vi "TI sbRIO Main (FPGA) old.vi"() -> ()   [LabVIEW 2019]
uses:
  <userlib>/_NI SPI IP/FPGA/Controllers/Public/Transfer Settings.ctl
  Type Defs/Diagnostic Mode.ctl
  Controls/SPI Channels.ctl
  <vilib>/Platform/TimedLoop/XDataNode/timing_clust.ctl
  <vilib>/Platform/TimedLoop/XDataNode/nitl_modes.ctl
  <vilib>/Platform/TimedLoop/XDataNode/wakeup.ctl
  <vilib>/rvi/FXPMathLib/FxpDiv/subVIs/nifxpmath_Div_SimConfig.ctl
  <vilib>/rvi/FXPMathLib/basic elements/FxpIntAccumulator/subVIs/nifxpmath_IntAccumulator_SimConfig.ctl
  <vilib>/rvi/FXPMathLib/FxpSqrt/subVIs/nifxpmath_Sqrt_SimConfig.ctl
  <vilib>/fxp/LVFixedPointOverflowPolicyTypeDef.ctl
  <userlib>/_NI SPI IP/FPGA/Controllers/Public/Spi Master Inputs.ctl
  <vilib>/rvi/Emulation/niFpgaGetClockAttributes.vi
  <vilib>/rvi/Emulation/niFpgaSctlEmulationGetInTimedLoop.vi
  <vilib>/rvi/Emulation/niFpgaEmulationReportErrorSimple.vi
  <vilib>/rvi/eio/common/nirviEmuTemplateMethod_errors.vi
  Onboard AIs Global.vi
  <vilib>/rvi/Emulation/niFpgaProcessEmulError.vi
  <vilib>/rvi/Emulation/niFpgaCriticalErrorInLSC.vi
  ADC AI Global.vi
  <vilib>/rvi/FXPMathLib/FxpDiv/simVIs/DllFxpDivTemp_sub.vi
  <vilib>/rvi/DataTransferAndStorage/Container/Common/niFpgaContainerExecOnDevCompGetState.vi
  <vilib>/rvi/Emulation/niFpgaEmulationIsFPGAContextNoSignature.vi
  <vilib>/rvi/errors/niFpgaSetErrorForExecOnDevCompSimple.vi
  <vilib>/rvi/eio/common/nirviEmuReportErrorAndStop.vi
  <vilib>/rvi/DataTransferAndStorage/Container/Common/niFpgaContainerGetUniqueNameForEmu.vi
  <vilib>/rvi/FIFO/Fifo_Resource/nirvififoEmulationSetSize.vi
  <vilib>/rvi/FIFO/Fifo_Resource/nirviFifoEmulationQueueMgr.vi
  <instcachedir>/0/nirviFifoEmulationQueueMgr_E5CAEC123FF24DC58D834DCA3CDAA9B5.lvgen/nirviFifoEmulationQueueMgr_E5CAEC123FF24DC58D834DCA3CDAA9B5_000.vi
  <vilib>/rvi/FIFO/Fifo_Resource/nirvififoEmulationDetermineInputValidOut.vi
  <vilib>/rvi/FIFO/Fifo_Resource/nirvififoEmulationCreateLock.vi
  <vilib>/rvi/FIFO/Fifo_Resource/nirvififoEmulationObtainLock.vi
  <vilib>/rvi/FIFO/Fifo_Resource/nirvififoEmulationReleaseLock.vi
  <vilib>/rvi/occurrence/nirviWaitOnOccurrenceBase.vi
  <vilib>/rvi/errors/nirviReportUnexpectedCaseInternalError.vi
  <vilib>/rvi/errors/nirviReportUnexpectedCaseInternalError (U32).vi
  <vilib>/Utility/error.llb/Clear Errors.vi
  <vilib>/rvi/interface/RandomDataEmulation/niFpgaRandomDataHandleErrors.vi
  Diagnostic Global.vi
  Diagnostic Global (U32).vi
  Flow Frequencies Global.vi
  ADC AI Global (Avg).vi
  <vilib>/rvi/Analysis/common/codeGenErrors/XNode/niFpgaXNodeCodeGenErrorHandle.vi
  <vilib>/rvi/FXPMathLib/basic elements/FxpIntAccumulator/simVIs/DllFxpIntAccumulator_sub.vi
  <vilib>/rvi/FXPMathLib/FxpSqrt/simVIs/DllSqrtTemp_sub.vi
  Pump Currents Global.vi
  ADC AI Global (U32).vi
  <vilib>/eio/EIONode/EIONode.xnode
  <vilib>/rvi/FXPMathLib/FxpDiv/XNode/nifxpmath_Div.xnode
  <vilib>/rvi/DataTransferAndStorage/Container/XNode/niFpgaContainer.xnode
  <vilib>/rvi/FIFO/Fifo_Resource/niFpgaFifoEmulationRefIn.vi
  <vilib>/rvi/FXPMathLib/FxpMul/XNode/nifxpmath_Multiplier.xnode
  <vilib>/rvi/FXPMathLib/FxpAdd/XNode/nifxpmath_Add.xnode
  <vilib>/rvi/Analysis/measure/butterworth/XNode/niFpgaButterworthFilter.xnode
  <vilib>/rvi/Analysis/measure/dc-rms/XNode/niFpgaDC-RMS.xnode
  <vilib>/Platform/TimedLoop/XDataNode/XDataNode.xnode
  <vilib>/rvi/FXPMathLib/basic elements/FxpIntAccumulator/XNode/nifxpmath_IntAccumulator.xnode
  <vilib>/rvi/FXPMathLib/FxpSqrt/XNode/nifxpmath_Sqrt.xnode
  <vilib>/eio/EIOMethodNode/EIOMethodNode.xnode
  <vilib>/rvi/interface/RandomDataEmulation/nirviRandomDataFpgaReadWriteTemplate.vi
  <vilib>/rvi/FXPMathLib/sim/FxpSim.dll
  <vilib>/Platform/TimedLoop/XDataNode/XDNodeRunTimeDep.lvlib
  <userlib>/_NI SPI IP/FPGA/Controllers/NI SPI IP FPGA.lvlib
panel:
  in  "PWM Freq":fxp<+,32,0>=2.499902620911598e-06 caption="frequency (periods/tick)"
  in  "PWM Duty":fxp<+,32,0>[](array[numeric])=[0.0, 0.0, 0.0, 0.0, 0.0, 0.0]
  out "Pump Cmds":fxp<+/-,28,17>[](array[numeric])
  in  "Pumps Present":bool[](array[boolean])=[FALSE, FALSE, FALSE, FALSE, FALSE, FALSE]
  in  "Pump Cmds (Duty)":u32[](array[numeric])=[0, 0, 0, 0, 0, 0]
  in  "Debug Restarts":bool
  out "Pump No Starts":u32[](array[numeric])
  in  "Initial No Starts":u32[](array[numeric])=[0, 0, 0, 0, 0, 0]
  in  "Pump Start Time":u32
  out "Restarts":i32[](array[numeric])
  out "Cmd Pump Starts":u32[](array[numeric])
  in  "Stop Command":fxp<+,32,0>
  in  "Initial Cmd Starts":u32[](array[numeric])=[0, 0, 0, 0, 0, 0]
  in  "Ctrl Currents":fxp<+/-,28,17>[](array[numeric])=[0.0, 0.0, 0.0, 0.0, 0.0, 0.0]
  in  "Initial Acutal Starts":u32[](array[numeric])=[0, 0, 0, 0, 0, 0]
  in  "Power Relays":bool[](array[boolean])=[FALSE, FALSE, FALSE, FALSE, FALSE, FALSE]
  out "Actual Pump Starts":u32[](array[numeric])
  out "Timers (ms)":u32[](array[numeric])
  out "Pump On States":bool[](array[boolean])
  in  "Off Current Thresh":fxp<+/-,28,17>
  in  "Min Off Time":u32
  in  "On Current Thresh":fxp<+/-,28,17>
  in  "Min On Time":u32
  in  "Reset Pump Starts":bool
  in  "Pump Starts Enable":bool
  in  "Diag Max Period (ticks)":u32
  in  "Diagnostic Mode":T1=enum."PSA"
  out "Elapsed Times OUT":fxp<+,40,40>[](array[numeric])
  out "Data OUT":fxp<+/-,28,17>[](array[numeric])
  in  "Diagnostic Filter":u16=5
  in  "Invert Diagnostic":bool
  in  "Diagnostic Freq Coeff":i32
  in  "Count Off-Time":bool
  in  "Elapsed Times":fxp<+,40,40>[](array[numeric])=[0.0, 0.0, 0.0, 0.0, 0.0, 0.0]
  in  "ADC Init":bool=TRUE
  in  "FFT_Amp?":bool=TRUE
  in  "Max Period (ticks)":u32
  in  "Freq Flow?":bool
  in  "Divide Value":u8=1
  in  "Current Threshold":fxp<+,26,7>=1.0 format="%#_22g"
  in  "Enable Timers":bool[](array[boolean])=[FALSE, FALSE, FALSE, FALSE, FALSE, FALSE]
  in  "PumpCurrentM":fxp<+/-,16,9>=-60.0 format="%#_25g"
  in  "PumpCurrentB":fxp<+/-,16,9>=-60.0 format="%#_25g"
  in  "InvertPWM?":bool
  in  "DIO25":bool
  in  "DIO24":bool
  out "DIO23":bool
  in  "DIO22":bool
  in  "DIO21":bool
  in  "DIO20":bool
  in  "DIO19":bool
  in  "DIO18":bool
  in  "DIO17":bool
  in  "DIO16":bool
  in  "DIO15":bool
  in  "DIO14":bool
  in  "DIO13":bool
  in  "DIO12":bool
  out "ADC Read Data":u64 format="%.0x"
  in  "ADC CS Mode":enum16{"All", "CS0", "CS1"}(ring)
  in  "ADC Trigger":bool=TRUE
  in  "ADC SPI Settings":T2 {"Direction Change Bit" max=64 step=1; "Transfer Length (bits)" min=1 max=64 step=1}
  in  "ADC Data In":u64 format="%.0x"
  in  "ADC Conversion Request":bool
  in  "ADC Manual":bool
  in  "Brushless":bool
  in  "AI Divisor":u32
  in  "AO3":fxp<+/-,20,5>
  in  "AO2":fxp<+/-,20,5>
  in  "Pressure Cmd":fxp<+/-,20,5>
  in  "PS Cmd":fxp<+/-,20,5>
  in  "Loop Timer (uSec)":u32=100
  in  "Timer Resets":bool[](array[boolean])=[FALSE, FALSE, FALSE, FALSE, FALSE, FALSE]
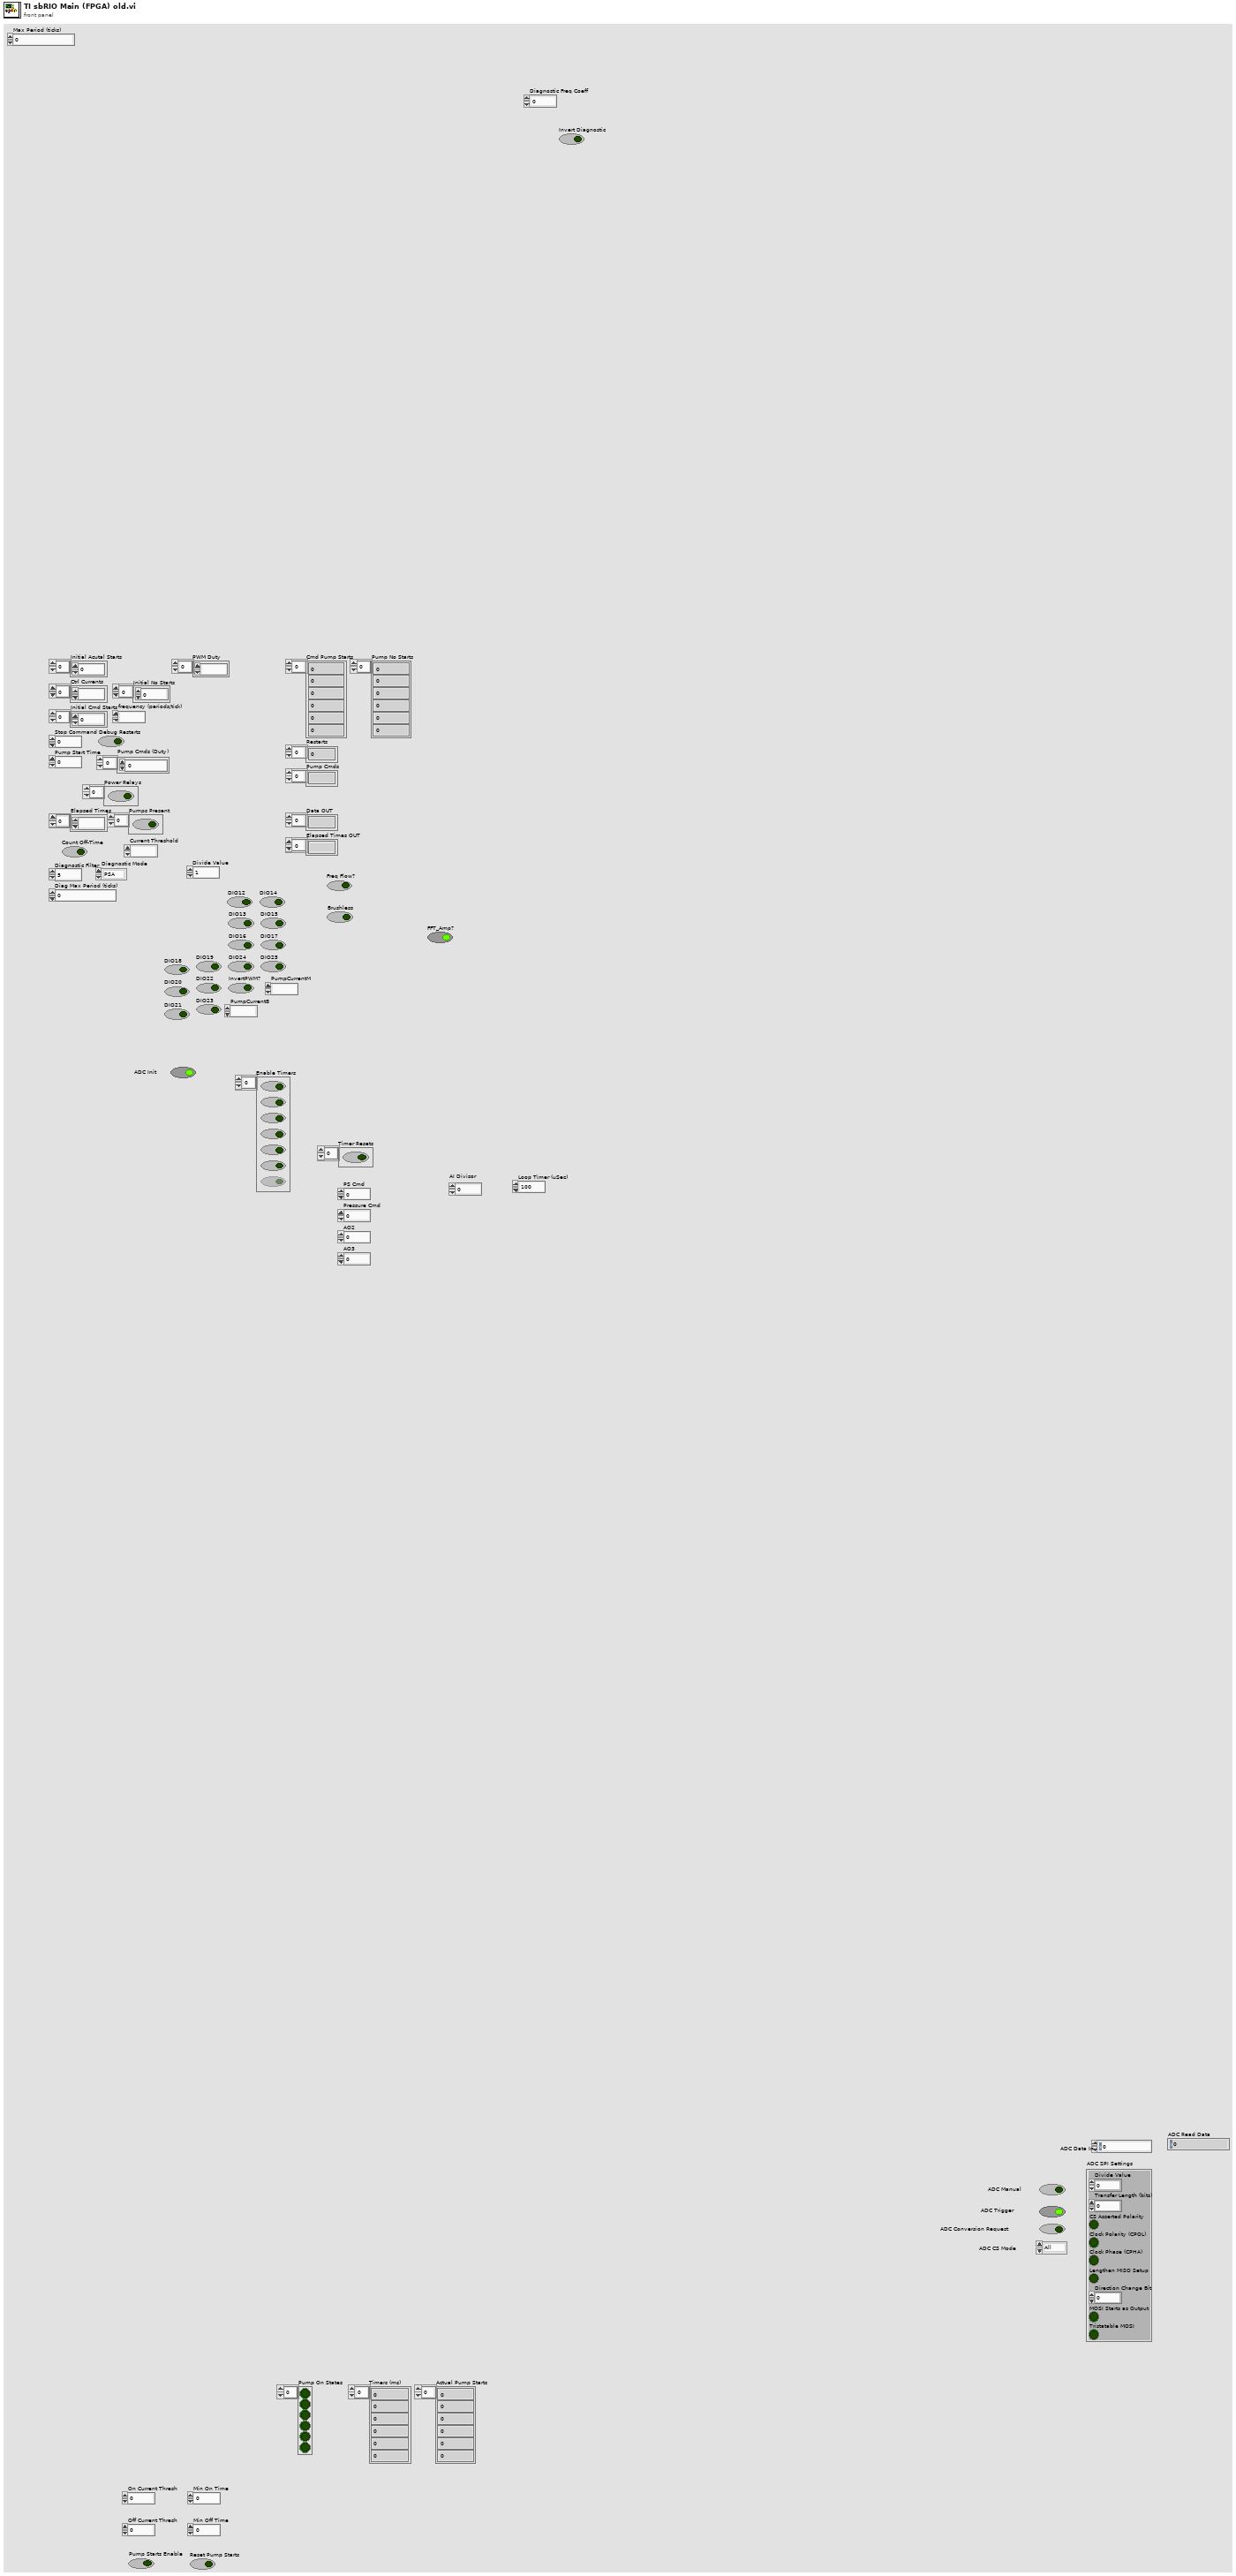
[diagram p1: front panel]
types:
  T1 = typedef "Diagnostic Mode.ctl" = enum16{"None", "PSA", "CMFB"}
  T2 = typedef "NI SPI IP FPGA.lvlib/Transfer Settings.ctl" = cluster{"Divide Value":u8, "Transfer Length (bits)":u8, "CS Asserted Polarity":bool, "Clock Polarity (CPOL)":bool, "Clock Phase (CPHA)":bool, "Lengthen MISO Setup":bool, "Direction Change Bit":u8, "MOSI Starts as Output":bool, "Tristatable MOSI":bool}
  T3 = typedef "SPI Channels.ctl" = cluster{"CS":refnum<k21>, "CLK":refnum<k21>, "MOSI":refnum<k21>, "MISO":refnum<k21>, "CONVST":refnum<k21>, "CDI":refnum<k21>, "CS1":refnum<k21>}
  T4 = typedef "XDNodeRunTimeDep.lvlib/timing_clust.ctl" = cluster{"Expected End [f-1]":u64, "Actual End [f-1]":u64, "Finished Late? [f-1]":bool, "Expected End [i-1]":u64, "Actual End [i-1]":u64, "Finished Late? [i-1]":bool, "Expected Start [i]":u64, "Actual Start [i]":u64, "Expected Start [f]":u64, "Actual Start [f]":u64, "Source Name":string, "Structure Name":string, "Period":i64, "Deadline":i64, "Offset":i64, "Start":i64, "Priority":i32, "Timeout":i32, "Mode":T5, "Wakeup Reason":T6, "Error":errorcluster, "Source Type":string, "Secondary Source Type":string, "Global End Time":u64, "Global Start Time":u64, "Frame Duration":u64, "Iteration Duration":u64, "Assigned CPU":i32, "I/O Scan Engine Mode":u32}
  T5 = typedef "XDNodeRunTimeDep.lvlib/nitl_modes.ctl" = enum32{"No Change", "Process missed periods, maintain original phase", "Discard missed periods, maintain original phase", "Process missed periods, ignore original phase", "Discard missed periods, ignore original phase"}
  T6 = typedef "XDNodeRunTimeDep.lvlib/wakeup.ctl" = enum32{"Normal", "Aborted", "Asynchronous wakeup", "Timing source error", "Timed loop error", "Timeout"}
  T7 = typedef "NI SPI IP FPGA.lvlib/Spi Master Inputs.ctl" = cluster{"MISO":bool}
  T8 = typedef "NI SPI IP FPGA.lvlib/Spi Master Outputs.ctl" = cluster{"Chip Select":bool, "Clock":bool, "MOSI":bool, "MOSI OE":bool}
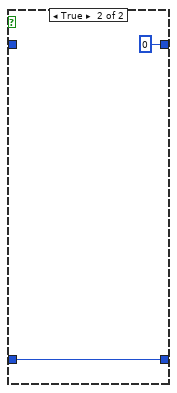
[diagram p3: hidden frame]
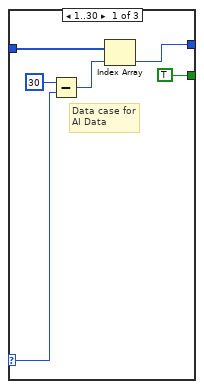
[diagram p6: hidden frame]
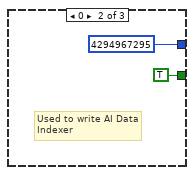
[diagram p7: hidden frame]
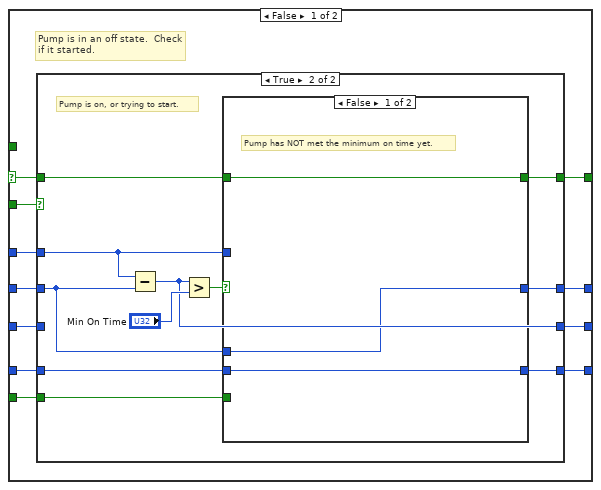
[diagram p13: hidden frame]
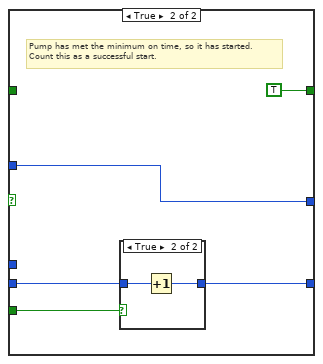
[diagram p15: hidden frame]
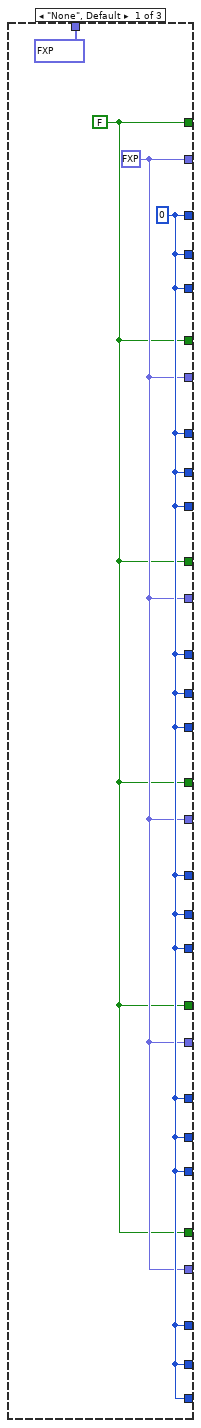
[diagram p20: hidden frame]
diagram:
  w34 = refnum<k21> "RMC/DIO60"  # CONVST
  w35 = refnum<k21> "RMC/DIO59"  # CDI
  w36 = refnum<k21> "RMC/DIO58"  # CS1
  # "Main source of data for RT."
  # "Pump Phase Current and Elapsed Times."
  # "PWM Outputs for Controller Command."
  # "Signal Averaging."
  # "FFT for Pump Speed."
  # "Pump Controller Diagnostics."
  # "Turbine Flow Meters."
  # "Control Signals"
  # "4x ADC\n\nAI16\tPump Current 1\nAI17\tPump Current 2\nAI18\tPump Current 3\nAI19\tPump Current 4\nAI20\tPump Current 5\nAI21\tPump Current 6\nAI22\tController Current 1\nAI23\tController Current 2\nAI24\tController Current 3\nAI25\tController Current 4\nAI26\tController Current 5\nAI27\tController Current 6\nAI28\tTemp 1\nAI29\tTemp 2\nAI30\tPump Pressure 1\nAI31\tPump Pressure 2\nAI32\tPump Pressure 3\nAI33\tPump Pressure 4\nAI34\tPump Pressure 5\nAI35\tPump Pressure 6\nAI36\tPump Flow 1\nAI37\tPump Flow 2\nAI38\tPump Flow 3\nAI39\tPump Flow 4\nAI40\tPump Flow 5\nAI41\tPump Flow 6\nAI42\tSpare\nAI43\tSpare\nAI44\tSpare\nAI45\tSpare\nAI46\tSpare\nAI47\tSpare"
  # "Onboard\n\nAI0/8\tVoltage 1\nAI1/9\tVoltage 2\nAI2/10\tVoltage 3\nAI3/11\tVoltage 4\nAI4/12\tVoltage 5\nAI5/13\tVoltage 6\nAI6\tSpare\nAI14\tSpare\nAI7\tSpare\nAI15\tPower Supply Sense"
  # "This code was created to use\nwith an 8ch analog input to SPI\nchip (ADS8332IPW)."
  # "Explanation for Rounding http://www.eetimes.com/document.asp?doc_id=1274485&page_number=1"
  # "Explanation of Saturation vs. wrapping:   http://www.mathworks.com/help/fixedpoint/ug/saturation-and-wrapping.html\n If scale is 0 to 8 and value is -2               Saturation: 0    Wrapping:  6"
  n1 = node-c288() -> (w2:T4)  [unwired: 1 in]
  n2 = node-c288() -> (w25:T4)  [unwired: 1 in]
  n3 = node-c288() -> (w23:T4)  [unwired: 1 in]
  n4 = disable-structure shown="FPGA_TARGET_CLASS==SBRIO_9627" {
    frame condition #0 (active) {
      w42 = bool[] [FALSE, FALSE, FALSE, FALSE, FALSE, FALSE]  # Pump Triggered
      w48 = bool[] [FALSE, FALSE, FALSE, FALSE, FALSE, FALSE]  # Pump On States
      # "Pump Start Monitor (for finding restarts)."
      n5 = call "Tick Count8"() -> ("Tick Count(mSec)"=w45:u32)
      n6 = local read "PWM Duty"() -> (w43:fxp<+,32,0>[])
      n7 = Initialize Array(w45, 6 ("dimension size")) -> (w41:u32[])
      n8 = while {
        shift-right: [w81] -> _
        shift-left: w41 -> [w84]
        shift-right: [w71] -> _
        shift-left: "Initial Acutal Starts" -> [w78]
        shift-right: [w82] -> _
        shift-left: w48 -> [w83]
        shift-right: [w80] -> _
        shift-left: _ -> [w79]
        shift-right: [w69] -> _
        shift-left: "Initial Cmd Starts" -> [w66]
        shift-right: [w72] -> _
        shift-left: w43 -> [w75]
        shift-right: [w64] -> _
        shift-left: w42 -> [w65]
        shift-right: [w63] -> _
        shift-left: w41 -> [w57]
        shift-right: [w61] -> _
        shift-left: "Initial No Starts" -> [w56]
        stop <- FALSE stop-if-true
        # "Pump Current\n(Flange-mount\nCtrl current)"
        n9 = local read "PWM Duty"() -> (w74:fxp<+,32,0>[])
        n10 = case shown="True" "Reset Pump Starts" {
          tunnel: w78 -> [w88 _]
          tunnel: [w88 w89] -> w76
          tunnel: [w87 w89] -> w67
          tunnel: w66 -> [w87 _]
          tunnel: [w86 w89] -> w55
          tunnel: w56 -> [w86 _]
          frame False {
          }
          frame True {
            w89 = u32[] [0, 0, 0, 0, 0, 0] ("Pump Starts")
            n11 = local write "Reset Pump Starts"(FALSE ("Reset Pump Starts")) -> ()
          }
        }
        n12 = global read "Pump Currents Global.vi" "Pump Currents"() -> (w49:fxp<+/-,28,17>[])
        n13 = Select(t="Ctrl Currents", s="Debug Restarts", f=w49) -> (s? t:f=w53:fxp<+/-,28,17>[])
        n14 = for {
          tunnel: w53 -> [w95] mode=indexing
          tunnel: w84 -> [w122] mode=indexing
          tunnel: w76 -> [w121] mode=indexing
          tunnel: [w120] -> w71 mode=indexing
          tunnel: w83 -> [w118] mode=indexing
          tunnel: [w119] -> w82 mode=indexing
          tunnel: [w117] -> w81 mode=indexing
          tunnel: [w116] -> w80 mode=indexing
          tunnel: w79 -> [w115] mode=indexing
          tunnel: w67 -> [w109] mode=indexing
          tunnel: w75 -> [w113] mode=indexing
          tunnel: w74 -> [w110] mode=indexing
          tunnel: "Stop Command" -> [w114]
          tunnel: [w108] -> w69 mode=indexing
          tunnel: [w110] -> w72 mode=indexing
          tunnel: w65 -> [w104] mode=indexing
          tunnel: [w101] -> w64 mode=indexing
          tunnel: [w105] -> w63 mode=indexing
          tunnel: w57 -> [w103] mode=indexing
          tunnel: "Pump Start Time" -> [w102]
          tunnel: w55 -> [w100] mode=indexing
          tunnel: [w99] -> w61 mode=indexing
          tunnel: "Pumps Present" -> [w93] mode=indexing
          tunnel: "Pump Starts Enable" -> [w92]
          n15 = And(x=w93, y=w92) -> (x .and. y?=w91:bool)
          n16 = call "Tick Count"() -> ("Tick Count(mSec)"=w107:u32)
          n17 = Less?(x=w95, y="Off Current Thresh") -> (x < y?=w96:bool)
          n18 = Greater?(x=w95, y="On Current Thresh") -> (0:w94:bool)
          n19 = Equal?(x=w114, y=w113) -> (x = y?=w112:bool)
          n20 = Not Equal?(x=w113, y=w110) -> (x != y?=w111:bool)
          n21 = Compound Arithmetic op=AND(w91, w112, w111) -> (w106:bool)
          n22 = case shown="True" w118 {
            selector: w118 -> [w161 w197]
            tunnel: w122 -> [w165 w201]
            tunnel: w121 -> [w164 w200]
            tunnel: [w163 w199] -> w120
            tunnel: [w162 w198] -> w119
            tunnel: w107 -> [w160 w196]
            tunnel: [w159 w195] -> w117
            tunnel: [w158 w194] -> w116
            tunnel: w115 -> [w157 w193]
            tunnel: w91 -> [w156 _]
            tunnel: w94 -> [w155 _]
            tunnel: w96 -> [_ w192]
            frame False {
              # "Pump is in an off state.  Check\nif it started."
              n23 = case shown="True" w155 {
                tunnel: w165 -> [_ w172]
                tunnel: w164 -> [w167 w178]
                tunnel: [w167 w177] -> w163
                tunnel: w161 -> [w169 w176]
                tunnel: [w169 w175] -> w162
                tunnel: w160 -> [w168 w173]
                tunnel: [w168 w174] -> w159
                tunnel: [w166 w171] -> w158
                tunnel: w157 -> [w166 _]
                tunnel: w156 -> [_ w170]
                frame False {
                  # "Pump is off."
                }
                frame True {
                  # "Pump is on, or trying to start."
                  n24 = Subtract(x=w173, y=w172) -> (x-y=w171:u32)
                  n25 = Greater?(x=w171, y="Min On Time") -> (0:w179:bool)
                  n26 = case shown="False" w179 {
                    tunnel: w178 -> [w183 w188]
                    tunnel: [w183 w187] -> w177
                    tunnel: w176 -> [w181 _]
                    tunnel: [w181 TRUE] -> w175
                    tunnel: [w182 w185] -> w174
                    tunnel: w173 -> [_ w185]
                    tunnel: w172 -> [w182 _]
                    tunnel: w170 -> [_ w184]
                    frame False {
                      # "Pump has NOT met the minimum on time yet."
                    }
                    frame True {
                      # "Pump has met the minimum on time, so it has started.\nCount this as a successful start."
                      n27 = case shown="True" w184 {
                        tunnel: w188 -> [w189 w191]
                        tunnel: [w189 w190] -> w187
                        frame False {
                        }
                        frame True {
                          n28 = Increment(x=w191) -> (x+1=w190:u32)
                        }
                      }
                    }
                  }
                }
              }
            }
            frame True {
              # "Pump is in an on state.  Check\nif it stopped."
              n29 = case shown="True" w192 {
                tunnel: w201 -> [_ w207]
                tunnel: w200 -> [w204 w213]
                tunnel: [w204 w212] -> w199
                tunnel: w197 -> [w203 w211]
                tunnel: [w203 w210] -> w198
                tunnel: w196 -> [w205 w208]
                tunnel: [w205 w209] -> w195
                tunnel: [w202 w206] -> w194
                tunnel: w193 -> [w202 _]
                frame False {
                  # "Pump is in on."
                }
                frame True {
                  # "Pump is off, but make sure it's\nacutally off, and not just noise.\nSo, check that current is low\nfor a minimum amount of time."
                  n30 = Subtract(x=w208, y=w207) -> (x-y=w206:u32)
                  n31 = Greater?(x=w206, y="Min Off Time") -> (0:w214:bool)
                  n32 = case shown="True" w214 {
                    tunnel: w213 -> [w217 w220]
                    tunnel: [w217 w220] -> w212
                    tunnel: w211 -> [w218 _]
                    tunnel: [w218 FALSE] -> w210
                    tunnel: [w216 w219] -> w209
                    tunnel: w208 -> [_ w219]
                    tunnel: w207 -> [w216 _]
                    frame False {
                      # "Pump has NOT met the minimum off time yet."
                    }
                    frame True {
                      # "Pump has met the minimum off time, so it is indeed off."
                    }
                  }
                }
              }
            }
          }
          n33 = case shown="True" w104 {
            selector: w104 -> [_ w129]
            tunnel: w109 -> [w126 w128]
            tunnel: [w126 w127] -> w108
            tunnel: w107 -> [w125 w135]
            tunnel: w106 -> [w124 _]
            tunnel: [w125 w136] -> w105
            tunnel: w103 -> [_ w130]
            tunnel: w102 -> [_ w139]
            tunnel: [w124 w134] -> w101
            tunnel: w100 -> [w123 w138]
            tunnel: [w123 w137] -> w99
            tunnel: w94 -> [_ w131]
            frame False {
            }
            frame True {
              n34 = Subtract(x=w135, y=w130) -> (x-y=w140:u32)
              n35 = Greater?(x=w140, y=w139) -> (0:w133:bool)
              n36 = Or(x=w131, y=w133) -> (x .or. y?=w132:bool)
              n37 = case shown="True" w132 {
                tunnel: w138 -> [w142 w151]
                tunnel: [w142 w150] -> w137
                tunnel: [w144 w149] -> w136
                tunnel: w135 -> [_ w149]
                tunnel: [w143 FALSE] -> w134
                tunnel: w131 -> [_ w147]
                tunnel: w130 -> [w144 _]
                tunnel: w129 -> [w143 _]
                tunnel: w128 -> [w141 w146]
                tunnel: [w141 w145] -> w127
                frame False {
                }
                frame True {
                  n38 = case shown="False" w147 {
                    tunnel: w151 -> [w153 w154]
                    tunnel: [w152 w154] -> w150
                    frame False {
                      n39 = Increment(x=w153) -> (x+1=w152:u32)
                    }
                    frame True {
                    }
                  }
                  n40 = Increment(x=w146) -> (x+1=w145:u32)
                }
              }
            }
          }
        }
        "Actual Pump Starts" <- w71
        "Timers (ms)" <- w80
        "Pump On States" <- w82
        "Cmd Pump Starts" <- w69
        "Pump No Starts" <- w61
        n41 = To Long Integer(number=w71) -> (32bit integer=w70:i32[])
        n42 = To Long Integer(number=w69) -> (32bit integer=w68:i32[])
        n43 = To Long Integer(number=w61) -> (32bit integer=w59:i32[])
        n44 = Subtract(x=w70, y=w68) -> (x-y=w60:i32[])
        n45 = Add(x=w60, y=w59) -> (x+y=→"Restarts":i32[])
      }
    }
    frame condition #1 {
    }
  }
  n46 = timed-loop {
    timing: w2 -> [_]
    timing-out: [_] -> w1
    stop <- FALSE stop-if-true
    n47 = Index Array(array="PWM Duty") -> (element #1=w227:fxp<+,32,0>, element #2=w226:fxp<+,32,0>, element #3=w225:fxp<+,32,0>, element #4=w224:fxp<+,32,0>, element #5=w223:fxp<+,32,0>, element #6=w222:fxp<+,32,0>)  [unwired: 6 in]
    n48 = call "Square Wave Generator"("frequency (periods/tick)"="PWM Freq", "duty cycle (periods)"=w227) -> ("square wave out"=w242:bool)  [unwired: 13 in]
    n49 = call "Square Wave Generator2"("frequency (periods/tick)"="PWM Freq", "duty cycle (periods)"=w226) -> ("square wave out"=w241:bool)  [unwired: 13 in]
    n50 = call "Square Wave Generator3"("frequency (periods/tick)"="PWM Freq", "duty cycle (periods)"=w225) -> ("square wave out"=w240:bool)  [unwired: 13 in]
    n51 = call "Square Wave Generator4"("frequency (periods/tick)"="PWM Freq", "duty cycle (periods)"=w224) -> ("square wave out"=w239:bool)  [unwired: 13 in]
    n52 = call "Square Wave Generator5"("frequency (periods/tick)"="PWM Freq", "duty cycle (periods)"=w223) -> ("square wave out"=w238:bool)  [unwired: 13 in]
    n53 = call "Square Wave Generator6"("frequency (periods/tick)"="PWM Freq", "duty cycle (periods)"=w222) -> ("square wave out"=w237:bool)  [unwired: 13 in]
    n54 = Exclusive Or(1:"InvertPWM?", 2:w242) -> (0:w235:bool)
    n55 = Exclusive Or(1:"InvertPWM?", 2:w241) -> (0:w234:bool)
    n56 = Exclusive Or(1:"InvertPWM?", 2:w240) -> (0:w233:bool)
    n57 = Exclusive Or(1:"InvertPWM?", 2:w239) -> (0:w232:bool)
    n58 = Exclusive Or(1:"InvertPWM?", 2:w238) -> (0:w231:bool)
    n59 = Exclusive Or(1:"InvertPWM?", 2:w237) -> (0:w230:bool)
    n60 = xnode "FPGA I/O Node"("RMC/DIO0"=w235, "RMC/DIO1"=w234, "RMC/DIO2"=w233, "RMC/DIO3"=w232, "RMC/DIO4"=w231, "RMC/DIO5"=w230) -> ()  [unwired: 7 in, 7 out]
  }
  n61 = Unbundle By Name(T3 {"CS"="RMC/DIO57", "CLK"="RMC/DIO54", "MOSI"="RMC/DIO56", "MISO"="RMC/DIO55", "CONVST"="RMC/DIO60", "CDI"="RMC/DIO59", "CS1"="RMC/DIO58"} ("SPI Channels")) -> ("CS"=w27:refnum<k21>, "CLK"=w28:refnum<k21>, "MOSI"=w29:refnum<k21>, "MISO"=w30:refnum<k21>)
  n62 = timed-loop {
    timing: w25 -> [_]
    timing-out: [_] -> w24
    stop <- FALSE stop-if-true
    n63 = Index Array(array="Power Relays") -> (element #1=w251:bool, element #2=w250:bool, element #3=w249:bool, element #4=w248:bool, element #5=w247:bool, element #6=w246:bool)  [unwired: 6 in]
    n64 = xnode "FPGA I/O Node"("RMC/DIO6"=w251, "RMC/DIO7"=w250, "RMC/DIO8"=w249, "RMC/DIO9"=w248, "RMC/DIO10"=w247, "RMC/DIO11"=w246, "RMC/DIO12"="DIO12", "RMC/DIO13"="DIO13", "RMC/DIO14"="DIO14", "RMC/DIO15"="DIO15", "RMC/DIO16"="DIO16", "RMC/DIO17"="DIO17", "RMC/DIO18"="DIO18", "RMC/DIO19"="DIO19", "RMC/DIO20"="DIO20", "RMC/DIO21"="DIO21", "RMC/DIO22"="DIO22", "RMC/DIO24"="DIO24", "RMC/DIO25"="DIO25") -> ("RMC/DIO23"=→"DIO23":bool)  [unwired: 21 in, 21 out]
  }
  n65 = timed-loop {
    timing: w23 -> [_]
    timing-out: [_] -> w22
    shift-right: [w394] -> _
    shift-left: u32 0 ("f") -> [w393]
    shift-right: [w276] -> _
    shift-left: fxp<+/-,28,17> 0.0 ("AI0") -> [w388]
    shift-right: [w363] -> _
    shift-left: u32 0 ("f") -> [w364]
    shift-right: [w275] -> _
    shift-left: fxp<+/-,28,17> 0.0 ("AI0") -> [w369]
    shift-right: [w354] -> _
    shift-left: u32 0 ("f") -> [w353]
    shift-right: [w274] -> _
    shift-left: fxp<+/-,28,17> 0.0 ("AI0") -> [w348]
    shift-right: [w323] -> _
    shift-left: u32 0 ("f") -> [w324]
    shift-right: [w273] -> _
    shift-left: fxp<+/-,28,17> 0.0 ("AI0") -> [w329]
    shift-right: [w314] -> _
    shift-left: u32 0 ("f") -> [w313]
    shift-right: [w272] -> _
    shift-left: fxp<+/-,28,17> 0.0 ("AI0") -> [w308]
    shift-right: [w283] -> _
    shift-left: u32 0 ("f") -> [w284]
    shift-right: [w271] -> _
    shift-left: fxp<+/-,28,17> 0.0 ("AI0") -> [w289]
    stop <- FALSE stop-if-true
    w278 = fxp<+,32,32> 40000000.0 ("x")
    n66 = xnode "FPGA I/O Node"() -> ("RMC/DIO32"=w398:bool)  [unwired: 1 in, 1 out]
    n67 = xnode "FPGA I/O Node"() -> ("RMC/DIO33"=w359:bool)  [unwired: 1 in, 1 out]
    n68 = xnode "FPGA I/O Node"() -> ("RMC/DIO34"=w358:bool)  [unwired: 1 in, 1 out]
    n69 = xnode "FPGA I/O Node"() -> ("RMC/DIO35"=w319:bool)  [unwired: 1 in, 1 out]
    n70 = xnode "FPGA I/O Node"() -> ("RMC/DIO36"=w318:bool)  [unwired: 1 in, 1 out]
    n71 = xnode "FPGA I/O Node"() -> ("RMC/DIO37"=w279:bool)  [unwired: 1 in, 1 out]
    n72 = feedback-in #1(w398) -> ()
    n73 = feedback #1() -> (w397:bool)  [unwired: 1 in]
    n74 = feedback #2() -> (w360:bool)  [unwired: 1 in]
    n75 = feedback-in #2(w359) -> ()
    n76 = feedback #3() -> (w357:bool)  [unwired: 1 in]
    n77 = feedback-in #3(w358) -> ()
    n78 = feedback #4() -> (w320:bool)  [unwired: 1 in]
    n79 = feedback-in #4(w319) -> ()
    n80 = feedback #5() -> (w317:bool)  [unwired: 1 in]
    n81 = feedback-in #5(w318) -> ()
    n82 = feedback #6() -> (w280:bool)  [unwired: 1 in]
    n83 = feedback-in #6(w279) -> ()
    n84 = Increment(x=w393) -> (x+1=w392:u32)
    n85 = Increment(x=w364) -> (x+1=w365:u32)
    n86 = Increment(x=w353) -> (x+1=w352:u32)
    n87 = Increment(x=w324) -> (x+1=w325:u32)
    n88 = Increment(x=w313) -> (x+1=w312:u32)
    n89 = Increment(x=w284) -> (x+1=w285:u32)
    n90 = Greater?(x=w398, y=w397) -> (0:w379:bool)
    n91 = Greater?(x=w359, y=w360) -> (0:w378:bool)
    n92 = Greater?(x=w358, y=w357) -> (0:w339:bool)
    n93 = Greater?(x=w319, y=w320) -> (0:w338:bool)
    n94 = Greater?(x=w318, y=w317) -> (0:w299:bool)
    n95 = Greater?(x=w279, y=w280) -> (0:w298:bool)
    n96 = Greater?(x=w392, y="Max Period (ticks)") -> (0:w396:bool)
    n97 = Greater?(x=w365, y="Max Period (ticks)") -> (0:w361:bool)
    n98 = Greater?(x=w352, y="Max Period (ticks)") -> (0:w356:bool)
    n99 = Greater?(x=w325, y="Max Period (ticks)") -> (0:w321:bool)
    n100 = Greater?(x=w312, y="Max Period (ticks)") -> (0:w316:bool)
    n101 = Greater?(x=w285, y="Max Period (ticks)") -> (0:w281:bool)
    n102 = To Fixed-Point(number=w392) -> (fixed-point=w391:fxp<+,32,32>)  [unwired: 1 in]
    n103 = To Fixed-Point(number=w365) -> (fixed-point=w366:fxp<+,32,32>)  [unwired: 1 in]
    n104 = To Fixed-Point(number=w352) -> (fixed-point=w351:fxp<+,32,32>)  [unwired: 1 in]
    n105 = To Fixed-Point(number=w325) -> (fixed-point=w326:fxp<+,32,32>)  [unwired: 1 in]
    n106 = To Fixed-Point(number=w312) -> (fixed-point=w311:fxp<+,32,32>)  [unwired: 1 in]
    n107 = To Fixed-Point(number=w285) -> (fixed-point=w286:fxp<+,32,32>)  [unwired: 1 in]
    n108 = feedback #7() -> (w380:bool)  [unwired: 1 in]
    n109 = And(x=w379, y=w380) -> (x .and. y?=w381:bool)
    n110 = feedback #8() -> (w377:bool)  [unwired: 1 in]
    n111 = And(x=w378, y=w377) -> (x .and. y?=w376:bool)
    n112 = feedback #9() -> (w340:bool)  [unwired: 1 in]
    n113 = And(x=w339, y=w340) -> (x .and. y?=w341:bool)
    n114 = feedback #10() -> (w337:bool)  [unwired: 1 in]
    n115 = And(x=w338, y=w337) -> (x .and. y?=w336:bool)
    n116 = feedback #11() -> (w300:bool)  [unwired: 1 in]
    n117 = And(x=w299, y=w300) -> (x .and. y?=w301:bool)
    n118 = feedback #12() -> (w297:bool)  [unwired: 1 in]
    n119 = And(x=w298, y=w297) -> (x .and. y?=w296:bool)
    n120 = xnode "High Throughput Divide"("x"=w278, "y"=w391, "input valid"=w381) -> ("x/y"=w387:fxp<+,28,17>, "output valid"=w383:bool, "ready for input"=w382:bool)  [unwired: 1 in]
    n121 = feedback-in #7(w382) -> ()
    n122 = xnode "High Throughput Divide"("x"=w278, "y"=w366, "input valid"=w376) -> ("x/y"=w370:fxp<+,28,17>, "output valid"=w374:bool, "ready for input"=w375:bool)  [unwired: 1 in]
    n123 = feedback-in #8(w375) -> ()
    n124 = xnode "High Throughput Divide"("x"=w278, "y"=w351, "input valid"=w341) -> ("x/y"=w347:fxp<+,28,17>, "output valid"=w343:bool, "ready for input"=w342:bool)  [unwired: 1 in]
    n125 = feedback-in #9(w342) -> ()
    n126 = xnode "High Throughput Divide"("x"=w278, "y"=w326, "input valid"=w336) -> ("x/y"=w330:fxp<+,28,17>, "output valid"=w334:bool, "ready for input"=w335:bool)  [unwired: 1 in]
    n127 = feedback-in #10(w335) -> ()
    n128 = xnode "High Throughput Divide"("x"=w278, "y"=w311, "input valid"=w301) -> ("x/y"=w307:fxp<+,28,17>, "output valid"=w303:bool, "ready for input"=w302:bool)  [unwired: 1 in]
    n129 = feedback-in #11(w302) -> ()
    n130 = xnode "High Throughput Divide"("x"=w278, "y"=w286, "input valid"=w296) -> ("x/y"=w290:fxp<+,28,17>, "output valid"=w294:bool, "ready for input"=w295:bool)  [unwired: 1 in]
    n131 = feedback-in #12(w295) -> ()
    n132 = Select(t=u32 0 ("f"), s=w383, f=w392) -> (s? t:f=w394:u32)
    n133 = Select(t=u32 0 ("f"), s=w374, f=w365) -> (s? t:f=w363:u32)
    n134 = Select(t=u32 0 ("f"), s=w343, f=w352) -> (s? t:f=w354:u32)
    n135 = Select(t=u32 0 ("f"), s=w334, f=w325) -> (s? t:f=w323:u32)
    n136 = Select(t=u32 0 ("f"), s=w303, f=w312) -> (s? t:f=w314:u32)
    n137 = Select(t=u32 0 ("f"), s=w294, f=w285) -> (s? t:f=w283:u32)
    n138 = To Fixed-Point(fixed-point type=fxp<+/-,28,17> 0.0 ("AI0"), number=w387) -> (fixed-point=w385:fxp<+/-,28,17>)
    n139 = To Fixed-Point(fixed-point type=fxp<+/-,28,17> 0.0 ("AI0"), number=w370) -> (fixed-point=w372:fxp<+/-,28,17>)
    n140 = To Fixed-Point(fixed-point type=fxp<+/-,28,17> 0.0 ("AI0"), number=w347) -> (fixed-point=w345:fxp<+/-,28,17>)
    n141 = To Fixed-Point(fixed-point type=fxp<+/-,28,17> 0.0 ("AI0"), number=w330) -> (fixed-point=w332:fxp<+/-,28,17>)
    n142 = To Fixed-Point(fixed-point type=fxp<+/-,28,17> 0.0 ("AI0"), number=w307) -> (fixed-point=w305:fxp<+/-,28,17>)
    n143 = To Fixed-Point(fixed-point type=fxp<+/-,28,17> 0.0 ("AI0"), number=w290) -> (fixed-point=w292:fxp<+/-,28,17>)
    n144 = Or(x=w396, y=w383) -> (x .or. y?=w389:bool)
    n145 = Or(x=w361, y=w374) -> (x .or. y?=w368:bool)
    n146 = Or(x=w356, y=w343) -> (x .or. y?=w349:bool)
    n147 = Or(x=w321, y=w334) -> (x .or. y?=w328:bool)
    n148 = Or(x=w316, y=w303) -> (x .or. y?=w309:bool)
    n149 = Or(x=w281, y=w294) -> (x .or. y?=w288:bool)
    n150 = Select(t=fxp<+/-,28,17> 0.0 ("AI0"), s=w396, f=w385) -> (s? t:f=w390:fxp<+/-,28,17>)
    n151 = Select(t=fxp<+/-,28,17> 0.0 ("AI0"), s=w361, f=w372) -> (s? t:f=w367:fxp<+/-,28,17>)
    n152 = Select(t=fxp<+/-,28,17> 0.0 ("AI0"), s=w356, f=w345) -> (s? t:f=w350:fxp<+/-,28,17>)
    n153 = Select(t=fxp<+/-,28,17> 0.0 ("AI0"), s=w321, f=w332) -> (s? t:f=w327:fxp<+/-,28,17>)
    n154 = Select(t=fxp<+/-,28,17> 0.0 ("AI0"), s=w316, f=w305) -> (s? t:f=w310:fxp<+/-,28,17>)
    n155 = Select(t=fxp<+/-,28,17> 0.0 ("AI0"), s=w281, f=w292) -> (s? t:f=w287:fxp<+/-,28,17>)
    n156 = Select(t=w390, s=w389, f=w388) -> (s? t:f=w276:fxp<+/-,28,17>)
    n157 = Select(t=w367, s=w368, f=w369) -> (s? t:f=w275:fxp<+/-,28,17>)
    n158 = Select(t=w350, s=w349, f=w348) -> (s? t:f=w274:fxp<+/-,28,17>)
    n159 = Select(t=w327, s=w328, f=w329) -> (s? t:f=w273:fxp<+/-,28,17>)
    n160 = Select(t=w310, s=w309, f=w308) -> (s? t:f=w272:fxp<+/-,28,17>)
    n161 = Select(t=w287, s=w288, f=w289) -> (s? t:f=w271:fxp<+/-,28,17>)
    n162 = Build Array(w276, w275, w274, w273, w272, w271) -> (w270:fxp<+/-,28,17>[])
    n163 = global write "Flow Frequencies Global.vi" "Flow Frequencies"(w270) -> ()
  }
  n164 = disable-structure shown="FPGA_TARGET_CLASS==SBRIO_9627" {
    frame condition #0 (active) {
      w576 = u8 31 ("Sample Divisor")
      # "DMA for crash files."
      n165 = node-c288() -> (w580:T4)  [unwired: 1 in]
      n166 = Decrement(x=w576) -> (x-1=w577:u8)
      n167 = timed-loop "AI Resample Loop" {
        timing: w580 -> [_]
        timing-out: [_] -> w579
        shift-right: [w603] -> _
        shift-left: u32 0 ("Sample Divisor") -> [w590]
        shift-right: [w602] -> _
        shift-left: w576 -> [w591]
        tunnel: w577 -> [w596]
        tunnel: w576 -> [w595]
        stop <- FALSE stop-if-true
        # "Press, Flow"
        # "Ctrlr Current"
        # "30 items"
        n168 = global read "ADC AI Global (U32).vi" "AI16-47 (U32)"() -> (w584:u32[])
        n169 = local read "Actual Pump Starts"() -> (w581:u32[])
        n170 = global read "Diagnostic Global (U32).vi" "Diag Global (U32)"() -> (w582:u32[])
        n171 = Less Or Equal?(x="AI Divisor", y=w590) -> (x <= y?=w594:bool)
        n172 = Array Subset(array=w584, length=6) -> (w586:u32[])  [unwired: 1 in]
        n173 = Array Subset(array=w584, index=14, length=6) -> (w585:u32[])
        n174 = Build Array (concatenate)(w586, w585, w581, w582, "Pump Cmds (Duty)") -> (w592:u32[])
        n175 = feedback #13() -> (w598:u32[])  [unwired: 1 in]
        n176 = Select(t=w592, s=w594, f=w598) -> (s? t:f=w597:u32[])
        n177 = feedback-in #13(w597) -> ()
        n178 = Less Or Equal?(x=w591, y=w596) -> (x <= y?=w600:bool)
        n179 = Or(x=w594, y=w600) -> (x .or. y?=w593:bool)
        n180 = case shown="True" w593 {
          tunnel: w591 -> [_ w612]
          tunnel: [w610 w613] -> w599
          tunnel: w597 -> [_ w611]
          tunnel: w595 -> [w610 _]
          frame False {
          }
          frame True {
            n181 = Decrement(x=w612) -> (x-1=w613:u8)
            n182 = case shown="Default" w613 {
              selector: w613 -> [w620 _ _]
              tunnel: [w618 u32 4294967295 ("AI0") u32 0 ("AI0")] -> w615
              tunnel: [TRUE TRUE FALSE] -> w614
              tunnel: w611 -> [w622 _ _]
              frame 1..30 {
                # "Data case for\nAI Data"
                n183 = Subtract(x=u8 30 ("Sample Divisor"), y=w620) -> (x-y=w619:u8)
                n184 = Index Array(array=w622, index=w619) -> (element=w618:u32)
              }
              frame 0 {
                # "Used to write AI Data\nIndexer"
              }
              frame Default {
                # "Sould never get to\nthis case."
              }
            }
            n185 = case shown="True" w614 {
              tunnel: w615 -> [_ w617]
              frame False {
              }
              frame True {
                n186 = xnode ("FIFO Method Node")("Element"=w617, "Timeout"=u8 0) -> ()  [unwired: 1 in, 2 out]
              }
            }
          }
        }
        n187 = case shown="False" w594 {
          tunnel: w590 -> [w607 _]
          tunnel: [w606 u32 0] -> w603
          tunnel: w599 -> [w605 w608]
          tunnel: [w605 w608] -> w602
          frame False {
            n188 = Increment(x=w607) -> (x+1=w606:u32)
          }
          frame True {
          }
        }
      }
      n189 = node-c288(w579) -> ()
    }
    frame condition #1 {
    }
  }
  n190 = while {
    shift-right: [w633] -> _
    shift-left: "Elapsed Times" -> [w644]
    shift-right: [w634] -> _
    shift-left: u32[] [0, 0, 0, 0, 0, 0] -> [w635]
    stop <- FALSE stop-if-true
    # "Pump Current\nAI16-21"
    # "from:S 64 44\nto: U 40 40"
    n191 = global read "ADC AI Global.vi" "AI16-47"() -> (w637:fxp<+/-,28,17>[])
    n192 = feedback #14() -> (w642:bool[])  [unwired: 1 in]
    n193 = feedback-in #14("Timer Resets") -> ()
    n194 = Array Subset(array=w637, index=0, length=6) -> (w639:fxp<+/-,28,17>[])
    n195 = Greater?(x="Timer Resets", y=w642) -> (0:w645:bool[])
    n196 = for {
      tunnel: w639 -> [w679] mode=indexing
      tunnel: w645 -> [w681] mode=indexing
      tunnel: [w651] -> w636 mode=indexing
      tunnel: w644 -> [w676] mode=indexing
      tunnel: [w675] -> w633 mode=indexing
      tunnel: "Enable Timers" -> [w670] mode=indexing
      tunnel: w635 -> [w658] mode=indexing
      tunnel: [w653] -> w634 mode=indexing
      tunnel: "Count Off-Time" -> [w649]
      i -> [w680]
      w674 = fxp<+/-,26,7> 0.0 ("out")
      # "Formerly looking for DC signal based on period detection\nNow looking for staying in the 0A range"
      # "Calibration issue should only\nbe if reading is negative at 0A"
      # "30ms calculated as longest waveform period"
      # "RMS vi only outputs positive values, so put back to negative if that's the way it went in.  This fixes a calibration issue."
      # "D2A factor"
      # "Rough scale and offset for\nspeed and RMS measurements."
      n197 = xnode "High Throughput Divide"("x"=w679, "y"=fxp<+,14,14> 13107.0 ("Current Scale")) -> ("x/y"=w673:fxp<+/-,28,17>)
      n198 = xnode ("High Throughput Multiply")("x"=w673, "y"="PumpCurrentM") -> ("x*y"=w672:fxp<+/-,29,10>)
      n199 = xnode ("High Throughput Add")("x"=w672, "y"="PumpCurrentB") -> ("x+y"=w661:fxp<+/-,30,11>)
      n200 = Less?(x=w661, y=fxp<+/-,30,11> 0.25) -> (x < y?=w659:bool)
      n201 = xnode "Butterworth Filter"("input data"=w661) -> ("output data"=w663:fxp<+/-,20,15>)  [unwired: 2 in, 1 out]
      n202 = case shown="True" w659 {
        tunnel: w658 -> [_ w684]
        tunnel: [u32 0 w683] -> w653
        frame False {
        }
        frame True {
          n203 = Increment(x=w684) -> (x+1=w683:u32)
        }
      }
      n204 = To Fixed-Point(fixed-point type=w674, number=w661) -> (fixed-point=w666:fxp<+/-,26,7>)
      n205 = To Fixed-Point(fixed-point type=w674, number=w663) -> (fixed-point=w664:fxp<+/-,26,7>)
      n206 = case shown="False" "Brushless" {
        tunnel: [w685 w686] -> w665
        tunnel: w666 -> [_ w686]
        tunnel: w664 -> [w685 _]
        frame False {
        }
        frame True {
        }
      }
      n207 = Greater?(x=w653, y=u32 300) -> (0:w654:bool)
      n208 = Less Than 0?(x=w665) -> (x < 0?=w657:bool)
      n209 = case shown="0, Default" w680 {
        tunnel: [w740 w850 w960 w1070 w1180 w1290] -> w667
        tunnel: w665 -> [w739 w849 w959 w1069 w1179 w1289]
        frame 0, Default {
          n210 = xnode ("DC and RMS Measurements 5")("input data"=w739) -> ("RMS"=w740:fxp<+,26,7>)  [unwired: 1 in, 1 out]
        }
        frame 1 {
          n211 = xnode ("DC and RMS Measurements")("input data"=w849) -> ("RMS"=w850:fxp<+,26,7>)  [unwired: 1 in, 1 out]
        }
        frame 2 {
          n212 = xnode ("DC and RMS Measurements 2")("input data"=w959) -> ("RMS"=w960:fxp<+,26,7>)  [unwired: 1 in, 1 out]
        }
        frame 3 {
          n213 = xnode ("DC and RMS Measurements 3")("input data"=w1069) -> ("RMS"=w1070:fxp<+,26,7>)  [unwired: 1 in, 1 out]
        }
        frame 4 {
          n214 = xnode ("DC and RMS Measurements 4")("input data"=w1179) -> ("RMS"=w1180:fxp<+,26,7>)  [unwired: 1 in, 1 out]
        }
        frame 5 {
          n215 = xnode ("DC and RMS Measurements 6")("input data"=w1289) -> ("RMS"=w1290:fxp<+,26,7>)  [unwired: 1 in, 1 out]
        }
      }
      n216 = And(x=w657, y=w654) -> (x .and. y?=w656:bool)
      n217 = To Fixed-Point(fixed-point type=fxp<+/-,28,17> 0.0 ("out"), number=w667) -> (fixed-point=w668:fxp<+/-,28,17>)
      n218 = case shown="True" w656 {
        tunnel: w668 -> [w687 w689]
        tunnel: [w687 w688] -> w651
        frame False {
        }
        frame True {
          n219 = Negate(x=w689) -> (-x=w688:fxp<+/-,29,18>)
        }
      }
      n220 = Greater?(x=w651, y="Current Threshold") -> (0:w650:bool)
      n221 = Or(x=w650, y=w649) -> (x .or. y?=w648:bool)
      n222 = case shown="True" w681 {
        tunnel: w648 -> [w720 _]
        tunnel: w676 -> [w719 _]
        tunnel: [w718 fxp<+,40,40> 0.0 ("AI0")] -> w675
        tunnel: w670 -> [w717 _]
        frame False {
          n223 = case shown="True" w717 {
            tunnel: w720 -> [_ w724]
            tunnel: w719 -> [w721 w723]
            tunnel: [w721 w722] -> w718
            frame False {
            }
            frame True {
              n224 = case shown="True" w724 {
                tunnel: [w725 w726] -> w722
                tunnel: w723 -> [w725 w728]
                frame False {
                }
                frame True {
                  # "Was: Sat/Trunc       Now:  Wrap/Trunc"
                  # "Greater than 1 amp, so pump is \"on\"."
                  n225 = xnode ("High Throughput Add")("x"=w728, "y"=fxp<+,1,1> 1.0) -> ("x+y"=w726:fxp<+,40,40>)
                }
              }
            }
          }
        }
        frame True {
        }
      }
    }
    n226 = call "Loop Timer"("Count(uSec)"="Loop Timer (uSec)") -> ()  [unwired: 1 out]
    n227 = global write "Pump Currents Global.vi" "Pump Currents"(w636) -> ()
    n228 = local write "Elapsed Times"(w633) -> ()
  }
  n229 = node-c288() -> (w38:T4)  [unwired: 1 in]
  n230 = node-c288() -> (w5:T4)  [unwired: 1 in]
  n231 = timed-loop "4x ADC SPI Loop" {
    shift-right: [w1423] -> _
    shift-left: fxp<+/-,28,17>[] [0.0, 0.0, 0.0, 0.0, 0.0, 0.0, 0.0, 0.0, 0.0, 0.0, 0.0, 0.0, 0.0, 0.0, 0.0, 0.0, 0.0, 0.0, 0.0, 0.0, 0.0, 0.0, 0.0, 0.0, 0.0, 0.0, 0.0, 0.0, 0.0, 0.0, 0.0, 0.0] -> [w1424]
    tunnel: w27 -> [w1422]
    tunnel: w28 -> [w1421]
    tunnel: w29 -> [w1420]
    tunnel: w30 -> [w1419]
    tunnel: w36 -> [w1418]
    tunnel: w34 -> [w1417]
    tunnel: w35 -> [w1416]
    timing: w38 -> [_]
    timing-out: [_] -> w37
    shift-right: [w1405] -> _
    shift-left: u8 2 ("lo(x)") -> [w1406]
    shift-right: [w1402] -> _
    shift-left: u8 0 ("lo(x)") -> [w1403]
    shift-right: [w1399] -> _
    shift-left: u32[] [0, 0, 0, 0, 0, 0, 0, 0, 0, 0, 0, 0, 0, 0, 0, 0, 0, 0, 0, 0, 0, 0, 0, 0, 0, 0, 0, 0, 0, 0, 0, 0] -> [w1400]
    stop <- FALSE stop-if-true
    n232 = flat-sequence {
      tunnel: [w1437] -> w1415
      tunnel: w1424 -> [w1437]
      tunnel: w1422 -> [w1436]
      tunnel: w1421 -> [w1435]
      tunnel: w1420 -> [w1434]
      tunnel: w1419 -> [w1433]
      tunnel: [w1436] -> w1414
      tunnel: [w1435] -> w1413
      tunnel: [w1434] -> w1412
      tunnel: [w1433] -> w1411
      tunnel: w1418 -> [w1432]
      tunnel: w1417 -> [w1431]
      tunnel: w1416 -> [w1430]
      tunnel: [w1432] -> w1410
      tunnel: [w1430] -> w1409
      tunnel: [w1431] -> w1408
      tunnel: [w1429] -> w1407
      tunnel: w1406 -> [w1429]
      tunnel: [w1428] -> w1404
      tunnel: w1403 -> [w1428]
      tunnel: [w1426] -> w1401
      tunnel: w1400 -> [w1426]
      tunnel: w1415 -> [w1482]
      tunnel: [w1481] -> w1423
      tunnel: w1414 -> [w1477]
      tunnel: w1413 -> [w1480]
      tunnel: w1412 -> [w1479]
      tunnel: w1411 -> [w1478]
      tunnel: w1410 -> [w1476]
      tunnel: w1409 -> [_]
      tunnel: w1408 -> [w1462]
      tunnel: w1407 -> [w1463]
      tunnel: [w1457] -> w1405
      tunnel: w1404 -> [w1456]
      tunnel: [w1455] -> w1402
      tunnel: w1401 -> [w1454]
      tunnel: [w1453] -> w1399
      frame #0 {
        # "Message Type Index"
        n233 = case shown="True" "ADC Init" {
          tunnel: w1436 -> [_ w1452]
          tunnel: w1435 -> [_ w1451]
          tunnel: w1434 -> [_ w1450]
          tunnel: w1433 -> [_ w1449]
          tunnel: w1432 -> [_ w1448]
          tunnel: w1431 -> [_ w1447]
          tunnel: w1430 -> [_ w1446]
          frame False {
          }
          frame True {
            w1439 = TRUE ("I/O Item")
            w1444 = TRUE ("Enable")
            n234 = xnode "FPGA I/O Method Node"("FPGA I/O In"=w1447, "Enable"=w1444) -> ("FPGA I/O Out"=w1440:refnum<k21>)
            n235 = xnode "FPGA I/O Method Node"("FPGA I/O In"=w1446, "Enable"=FALSE) -> ()  [unwired: 1 out]
            n236 = xnode "FPGA I/O Method Node"("FPGA I/O In"=w1448, "Enable"=w1444) -> ("FPGA I/O Out"=w1443:refnum<k21>)
            n237 = xnode "FPGA I/O Method Node"("FPGA I/O In"=w1452, "Enable"=w1444) -> ("FPGA I/O Out"=w1442:refnum<k21>)
            n238 = xnode "FPGA I/O Method Node"("FPGA I/O In"=w1451, "Enable"=w1444) -> ()  [unwired: 1 out]
            n239 = xnode "FPGA I/O Method Node"("FPGA I/O In"=w1450, "Enable"=w1444) -> ()  [unwired: 1 out]
            n240 = xnode "FPGA I/O Method Node"("FPGA I/O In"=w1449, "Enable"=FALSE) -> ()  [unwired: 1 out]
            n241 = xnode "FPGA I/O Node"("I/O Item"=w1439, "FPGA I/O In"=w1440, "I/O Item"=w1439, "FPGA I/O In"=w1443, "I/O Item"=w1439, "FPGA I/O In"=w1442) -> ()  [unwired: 3 out]
            n242 = local write "ADC Init"(FALSE ("ADC Init")) -> ()
          }
        }
      }
      frame #1 {
        # "Message Index"
        # "Channel Index"
        # "16 Bits-Send Channel Selection, CS Normal \n42 Bits Assert Conversion Request, CS Not Enabled\n64 Bits - Unassert Conversion, CS Normal"
        # "CONVERSION REQ"
        n243 = xnode "FPGA I/O Node"("FPGA I/O In"=w1478) -> ("I/O Item"=w1483:bool)  [unwired: 1 out]
        n244 = Bundle By Name(cluster=T7 {"MISO"=FALSE} ("spi input"), "MISO"=w1483) -> (w1484:T7)
        n245 = feedback #15(TRUE ("Chip Select")) -> (w1459:bool)
        n246 = case shown="True" "ADC Manual" {
          tunnel: w1459 -> [w1491 w1544]
          tunnel: [w1491 w1543] -> w1465
          tunnel: [w1496 "ADC SPI Settings"] -> w1464
          tunnel: w1463 -> [w1490 _]
          tunnel: [w1492 "ADC Data In"] -> w1460
          tunnel: [w1489 w1539] -> w1457
          tunnel: [w1495 "ADC Conversion Request"] -> w1461
          tunnel: w1456 -> [w1494 _]
          tunnel: [w1493 w1539] -> w1455
          frame False {
            # "Auto Mode"
            n247 = Boolean To (0,1)(Boolean=w1491) -> (0, 1=w1503:i16)
            n248 = To Unsigned Byte Integer(number=w1503) -> (unsigned 8bit integer=w1502:u8)
            n249 = Add(x=w1502, y=w1490) -> (x+y=w1498:u8)
            n250 = Greater?(x=w1498, y=u8 2) -> (0:w1500:bool)
            n251 = Select(t=u8 0 ("y"), s=w1500, f=w1498) -> (s? t:f=w1497:u8)
            n252 = case shown="2" w1497 {
              selector: w1497 -> [w1510 w1516 w1526]
              tunnel: [w1504 w1513 w1520] -> w1496
              tunnel: [TRUE ("I/O Item") FALSE ("I/O Item") TRUE ("I/O Item")] -> w1495
              tunnel: w1494 -> [w1509 w1517 w1525]
              tunnel: [w1509 w1517 w1524] -> w1493
              tunnel: [w1507 u64 0 u64 53248] -> w1492
              tunnel: w1491 -> [_ _ w1528]
              tunnel: w1490 -> [_ _ w1523]
              tunnel: [w1510 w1516 w1527] -> w1489
              tunnel: "Divide Value" -> [w1505 w1515 w1522]
              frame 0, Default {
                # "16 Bits"
                # "Channel Select"
                # "0x#000"
                n253 = Bundle By Name(cluster=T2 {"Divide Value"=1, "Transfer Length (bits)"=16, "CS Asserted Polarity"=FALSE, "Clock Polarity (CPOL)"=TRUE, "Clock Phase (CPHA)"=FALSE, "Lengthen MISO Setup"=FALSE, "Direction Change Bit"=0, "MOSI Starts as Output"=FALSE, "Tristatable MOSI"=FALSE} ("Master Settings 2"), "Divide Value"=w1505) -> (w1504:T2)
                n254 = To Unsigned Quad Integer(1:w1509) -> (0:w1508:u64)
                n255 = Logical Shift(y=i16 12, x=w1508) -> (x << y=w1507:u64)
              }
              frame 1 {
                # "Conversion Request Asserted"
                # "42 Bits"
                # "Dont Care"
                n256 = Bundle By Name(cluster=T2 {"Divide Value"=1, "Transfer Length (bits)"=42, "CS Asserted Polarity"=FALSE, "Clock Polarity (CPOL)"=TRUE, "Clock Phase (CPHA)"=FALSE, "Lengthen MISO Setup"=FALSE, "Direction Change Bit"=0, "MOSI Starts as Output"=FALSE, "Tristatable MOSI"=FALSE} ("Master Settings 2"), "Divide Value"=w1515) -> (w1513:T2)
              }
              frame 2 {
                # "64 Bits"
                # "Read CMD"
                n257 = Bundle By Name(cluster=T2 {"Divide Value"=1, "Transfer Length (bits)"=64, "CS Asserted Polarity"=FALSE, "Clock Polarity (CPOL)"=TRUE, "Clock Phase (CPHA)"=FALSE, "Lengthen MISO Setup"=FALSE, "Direction Change Bit"=0, "MOSI Starts as Output"=FALSE, "Tristatable MOSI"=FALSE} ("Master Settings 2"), "Divide Value"=w1522) -> (w1520:T2)
                n258 = case shown="False" w1528 {
                  tunnel: [w1531 w1535] -> w1527
                  tunnel: w1526 -> [_ w1535]
                  tunnel: w1525 -> [w1532 w1536]
                  tunnel: [w1532 w1533] -> w1524
                  tunnel: w1523 -> [w1531 _]
                  frame False {
                  }
                  frame True {
                    n259 = Increment(x=w1536) -> (x+1=w1534:u8)
                    n260 = case shown="8" w1534 {
                      selector: w1534 -> [w1537 _]
                      tunnel: [w1537 u8 0] -> w1533
                      frame Default {
                      }
                      frame 8 {
                      }
                    }
                  }
                }
              }
            }
          }
          frame True {
            w1539 = u8 0 ("y")
            # "Manual Mode"
            n261 = feedback #16(FALSE) -> (w1548:bool)
            n262 = feedback-in #16("ADC Trigger") -> ()
            n263 = Greater?(x="ADC Trigger", y=w1548) -> (0:w1545:bool)
            n264 = And(x=w1545, y=w1544) -> (x .and. y?=w1543:bool)
          }
        }
        n265 = call <userlib>:"Spi Master.vi"("spi input"=w1484, "start strobe"=w1465, "data to write"=w1460, "MOSI output enable done"=TRUE, "spi transfer settings"=w1464) -> ("spi output"=w1487:T8, "read data valid"=w1458:bool, "read data"=w1472:u64, "ready for input"=w1474:bool)  [unwired: 7 in]
        "ADC Read Data" <- w1472
        n266 = feedback-in #15(w1474) -> ()
        n267 = Unbundle By Name(w1487) -> ("Chip Select"=w1469:bool, "Clock"=w1473:bool, "MOSI"=w1486:bool)
        n268 = case shown="\"All\", Default" "ADC CS Mode" {
          tunnel: w1469 -> [w1550 w1552 w1556]
          tunnel: [TRUE ("Chip Select") w1552 w1555] -> w1468
          tunnel: [w1550 TRUE ("Chip Select") w1554] -> w1467
          tunnel: w1457 -> [_ _ w1558]
          frame "CS1" {
          }
          frame "CS0" {
          }
          frame "All", Default {
            n269 = Equal?(x=w1558, y=u8 1) -> (x = y?=w1553:bool)
            n270 = case shown="True" w1553 {
              tunnel: w1556 -> [w1559 _]
              tunnel: [w1559 w1560] -> w1555
              tunnel: [w1559 w1560] -> w1554
              frame False {
              }
              frame True {
                w1560 = TRUE ("Chip Select")
              }
            }
          }
        }
        n271 = case shown="True" w1458 {
          tunnel: w1472 -> [_ w1569]
          tunnel: w1482 -> [w1562 w1568]
          tunnel: [w1562 w1567] -> w1481
          tunnel: w1460 -> [_ w1566]
          tunnel: w1455 -> [_ w1565]
          tunnel: w1454 -> [w1561 w1564]
          tunnel: [w1561 w1563] -> w1453
          frame False {
          }
          frame True {
            n272 = case shown="53248" w1566 {
              tunnel: w1569 -> [_ w1600]
              tunnel: w1568 -> [w1571 w1599]
              tunnel: [w1571 w1586] -> w1567
              tunnel: w1565 -> [_ w1592]
              tunnel: w1564 -> [w1570 w1585]
              tunnel: [w1570 w1576] -> w1563
              frame Default {
              }
              frame 53248 {
                w1591 = fxp<+/-,28,17> 0.0 ("AI0")
                # "0xD000"
                n273 = case shown="Default" w1592 {
                  selector: w1592 -> [w1601 _]
                  tunnel: [w1602 u8 7] -> w1593
                  frame Default {
                    n274 = Decrement(x=w1601) -> (x-1=w1602:u8)
                  }
                  frame 0 {
                  }
                }
                n275 = Split Number(x=w1600) -> (hi(x)=w1598:u32, lo(x)=w1597:u32)
                n276 = To Long Integer(number=w1593) -> (32bit integer=w1584:i32)
                n277 = Split Number(x=w1598) -> (hi(x)=w1577:u16, lo(x)=w1579:u16)
                n278 = Split Number(x=w1597) -> (hi(x)=w1580:u16, lo(x)=w1581:u16)
                n279 = To Unsigned Long Integer(number=w1581) -> (unsigned 32bit integer=w1575:u32)
                n280 = To Unsigned Long Integer(number=w1580) -> (unsigned 32bit integer=w1574:u32)
                n281 = To Unsigned Long Integer(number=w1579) -> (unsigned 32bit integer=w1573:u32)
                n282 = To Unsigned Long Integer(number=w1577) -> (unsigned 32bit integer=w1572:u32)
                n283 = To Fixed-Point(fixed-point type=w1591, number=w1577) -> (fixed-point=w1587:fxp<+/-,28,17>)
                n284 = To Fixed-Point(fixed-point type=w1591, number=w1579) -> (fixed-point=w1588:fxp<+/-,28,17>)
                n285 = To Fixed-Point(fixed-point type=w1591, number=w1580) -> (fixed-point=w1589:fxp<+/-,28,17>)
                n286 = To Fixed-Point(fixed-point type=w1591, number=w1581) -> (fixed-point=w1590:fxp<+/-,28,17>)
                n287 = Add(x=w1584, y=8) -> (x+y=w1583:i32)
                n288 = Add(x=w1584, y=16) -> (x+y=w1582:i32)
                n289 = Add(x=w1584, y=24) -> (x+y=w1578:i32)
                n290 = Replace Array Subset(array=w1599, new element #1=w1590, index #1=w1584, new element #2=w1589, index #2=w1583, new element #3=w1588, index #3=w1582, new element #4=w1587, index #4=w1578) -> (w1586:fxp<+/-,28,17>[])
                n291 = Replace Array Subset(array=w1585, new element #1=w1575, index #1=w1584, new element #2=w1574, index #2=w1583, new element #3=w1573, index #3=w1582, new element #4=w1572, index #4=w1578) -> (w1576:u32[])
                n292 = global write "ADC AI Global (U32).vi" "AI16-47 (U32)"(w1576) -> ()
                n293 = global write "ADC AI Global.vi" "AI16-47"(w1586) -> ()
              }
            }
          }
        }
        n294 = xnode "FPGA I/O Node"("I/O Item"=w1467, "FPGA I/O In"=w1476, "I/O Item"=w1468, "FPGA I/O In"=w1477, "I/O Item"=w1473, "FPGA I/O In"=w1480, "I/O Item"=w1486, "FPGA I/O In"=w1479, "I/O Item"=w1461, "FPGA I/O In"=w1462) -> ()  [unwired: 5 out]
      }
    }
  }
  n295 = timed-loop {
    timing: w5 -> [_]
    timing-out: [_] -> w4
    stop <- FALSE stop-if-true
    w1606 = fxp<+/-,28,17>[] [0.0, 0.0, 0.0, 0.0, 0.0, 0.0]  # Speed Placeholder
    n296 = global read "Pump Currents Global.vi" "Pump Currents"() -> (w1611:fxp<+/-,28,17>[])
    n297 = global read "ADC AI Global (Avg).vi" "AI22-47 (Avg)"() -> (w1610:fxp<+/-,28,17>[])
    n298 = local read "Elapsed Times"() -> (→"Elapsed Times OUT":fxp<+,40,40>[])
    n299 = global read "Onboard AIs Global.vi" "Onboard AI's"() -> (w1609:fxp<+/-,28,17>[])
    n300 = global read "Diagnostic Global.vi" "Diag_Global"() -> (w1612:fxp<+/-,28,17>[])
    n301 = Build Array (concatenate)(w1609, w1611, w1606, w1610, w1612) -> (→"Data OUT":fxp<+/-,28,17>[])
  }
  n302 = node-c288(w24) -> ()
  n303 = while {
    stop <- FALSE stop-if-true
    n304 = xnode "FPGA I/O Node"("AO0"="PS Cmd", "AO1"="Pressure Cmd", "AO2"="AO2", "AO3"="AO3") -> ()  [unwired: 5 in, 5 out]
  }
  n305 = while {
    stop <- FALSE stop-if-true
    w1628 = fxp<+/-,28,17> 0.0 ("Controller_Current_1 (AI6)")
    # "set at 100 Hz"
    # "S 28 17"
    # "S 24 5"
    n306 = xnode "FPGA I/O Node"() -> ("Voltage_1 (AI0/8)"=w1634:fxp<+/-,24,5>, "Voltage_2 (AI1/9)"=w1630:fxp<+/-,24,5>, "Voltage_3 (AI2/10)"=w1631:fxp<+/-,24,5>, "Voltage_4 (AI3/11)"=w1629:fxp<+/-,24,5>, "Voltage_5 (AI4/12)"=w1632:fxp<+/-,24,5>, "Voltage_6 (AI5/13)"=w1633:fxp<+/-,24,5>, "Spare_1"=w1641:fxp<+/-,24,5>, "Spare_2"=w1642:fxp<+/-,24,5>, "Spare_3"=w1643:fxp<+/-,24,5>, "PS_Sense (AI15)"=w1644:fxp<+/-,24,5>)  [unwired: 10 in, 10 out]
    n307 = To Fixed-Point(fixed-point type=w1628, number=w1634) -> (fixed-point=w1627:fxp<+/-,28,17>)
    n308 = To Fixed-Point(fixed-point type=w1628, number=w1630) -> (fixed-point=w1626:fxp<+/-,28,17>)
    n309 = To Fixed-Point(fixed-point type=w1628, number=w1631) -> (fixed-point=w1625:fxp<+/-,28,17>)
    n310 = To Fixed-Point(fixed-point type=w1628, number=w1629) -> (fixed-point=w1623:fxp<+/-,28,17>)
    n311 = To Fixed-Point(fixed-point type=w1628, number=w1632) -> (fixed-point=w1622:fxp<+/-,28,17>)
    n312 = To Fixed-Point(fixed-point type=w1628, number=w1633) -> (fixed-point=w1621:fxp<+/-,28,17>)
    n313 = To Fixed-Point(fixed-point type=w1628, number=w1641) -> (fixed-point=w1636:fxp<+/-,28,17>)
    n314 = To Fixed-Point(fixed-point type=w1628, number=w1642) -> (fixed-point=w1637:fxp<+/-,28,17>)
    n315 = To Fixed-Point(fixed-point type=w1628, number=w1643) -> (fixed-point=w1638:fxp<+/-,28,17>)
    n316 = To Fixed-Point(fixed-point type=w1628, number=w1644) -> (fixed-point=w1639:fxp<+/-,28,17>)
    n317 = Build Array(w1627, w1626, w1625, w1623, w1622, w1621, w1636, w1637, w1638, w1639) -> (w1624:fxp<+/-,28,17>[])
    n318 = global write "Onboard AIs Global.vi" "Onboard AI's"(w1624) -> ()
    n319 = call "Wait"("Count(mSec)"=u32 10) -> ()  [unwired: 1 out]
  }
  n320 = node-c288(w1) -> ()
  n321 = node-c288(w4) -> ()
  n322 = while {
    shift-right: [w1655] -> _
    shift-left: 0 ("Moving Point Index") -> [w1656]
    stop <- FALSE stop-if-true
    w1654 = 127 ("N (# of Ave Pts 8 max)")
    # "Ctrl Current, Temp,\nPressure, Flow\nAI22-47"
    # "S 28 17"
    # "set at 1 kHz"
    n323 = global read "Flow Frequencies Global.vi" "Flow Frequencies"() -> (w1645:fxp<+/-,28,17>[])
    n324 = global read "ADC AI Global.vi" "AI16-47"() -> (w1650:fxp<+/-,28,17>[])
    n325 = Array Subset(array=w1650, index=6, length=26) -> (w1647:fxp<+/-,28,17>[])
    n326 = case shown="True" "Freq Flow?" {
      tunnel: w1647 -> [w1662 w1666]
      tunnel: w1645 -> [_ w1665]
      tunnel: [w1662 w1663] -> w1646
      frame False {
      }
      frame True {
        n327 = Replace Array Subset(array=w1666, new element=w1665, index=14) -> (w1663:fxp<+/-,28,17>[])
      }
    }
    n328 = for {
      tunnel: w1656 -> [w1667]
      tunnel: w1654 -> [w1668]
      tunnel: [w1672] -> w1649 mode=indexing
      tunnel: w1646 -> [w1671] mode=indexing
      tunnel: refnum<k21> "Running Avg Memory" ("Memory") -> [w1670]
      i -> [w1669]
      n329 = call "Moving Average.vi"("Memory In"=w1670, "N (# of Ave Pts 127 max)"=w1668, "Moving Point Index"=w1667, "Data IN"=w1671, "Channel#"=w1669) -> ("Averaged Data"=w1672:fxp<+/-,28,17>)  [unwired: 10 in]
    }
    n330 = global write "ADC AI Global (Avg).vi" "AI22-47 (Avg)"(w1649) -> ()
    n331 = Increment(x=w1656) -> (x+1=w1658:i32)
    n332 = Greater Or Equal?(x=w1656, y=w1654) -> (x >= y?=w1657:bool)
    n333 = Select(t=0, s=w1657, f=w1658) -> (s? t:f=w1655:i32)
    n334 = call "Wait2"("Count(mSec)"=u32 1) -> ()  [unwired: 1 out]
  }
  n335 = disable-structure shown="FPGA_TARGET_CLASS==SBRIO_9627" {
    frame condition #0 (active) {
      n336 = while {
        stop <- FALSE stop-if-true
        n337 = local read "Pump Cmds (Duty)"() -> (w1674:u32[])
        n338 = for {
          tunnel: w1674 -> [w1677] mode=indexing
          tunnel: [w1676] -> w1673 mode=indexing
          n339 = To Fixed-Point(fixed-point type=fxp<+/-,28,17> 0.0 ("AI0"), number=w1677) -> (fixed-point=w1676:fxp<+/-,28,17>)
        }
        "Pump Cmds" <- w1673
      }
    }
    frame condition #1 {
    }
  }
  n340 = node-c288(w22) -> ()
  n341 = node-c288() -> (w7:T4)  [unwired: 1 in]
  n342 = timed-loop {
    shift-right: [w1758] -> _
    shift-left: _ -> [w1757]
    shift-right: [w1756] -> _
    shift-left: _ -> [w1755]
    shift-right: [w1753] -> _
    shift-left: _ -> [w1754]
    shift-right: [w1751] -> _
    shift-left: _ -> [w1752]
    timing: w7 -> [_]
    timing-out: [_] -> w6
    shift-right: [w1749] -> _
    shift-left: _ -> [w1750]
    shift-right: [w1740] -> _
    shift-left: _ -> [w1741]
    shift-right: [w1742] -> _
    shift-left: _ -> [w1743]
    shift-right: [w1745] -> _
    shift-left: _ -> [w1744]
    shift-right: [w1747] -> _
    shift-left: _ -> [w1746]
    shift-right: [w1703] -> _
    shift-left: _ -> [w1748]
    shift-right: [w1739] -> _
    shift-left: _ -> [w1738]
    shift-right: [w1737] -> _
    shift-left: _ -> [w1736]
    shift-right: [w1734] -> _
    shift-left: _ -> [w1735]
    shift-right: [w1732] -> _
    shift-left: _ -> [w1733]
    shift-right: [w1702] -> _
    shift-left: _ -> [w1731]
    shift-right: [w1722] -> _
    shift-left: _ -> [w1723]
    shift-right: [w1724] -> _
    shift-left: _ -> [w1725]
    shift-right: [w1727] -> _
    shift-left: _ -> [w1726]
    shift-right: [w1729] -> _
    shift-left: _ -> [w1728]
    shift-right: [w1701] -> _
    shift-left: _ -> [w1730]
    shift-right: [w1721] -> _
    shift-left: _ -> [w1720]
    shift-right: [w1719] -> _
    shift-left: _ -> [w1718]
    shift-right: [w1716] -> _
    shift-left: _ -> [w1717]
    shift-right: [w1714] -> _
    shift-left: _ -> [w1715]
    shift-right: [w1700] -> _
    shift-left: _ -> [w1713]
    shift-right: [w1704] -> _
    shift-left: _ -> [w1705]
    shift-right: [w1706] -> _
    shift-left: _ -> [w1707]
    shift-right: [w1709] -> _
    shift-left: _ -> [w1708]
    shift-right: [w1711] -> _
    shift-left: _ -> [w1710]
    shift-right: [w1699] -> _
    shift-left: _ -> [w1712]
    stop <- FALSE stop-if-true
    n343 = xnode "FPGA I/O Node"() -> ("RMC/DIO38"=w1679:bool)  [unwired: 1 in, 1 out]
    n344 = xnode "FPGA I/O Node"() -> ("RMC/DIO39"=w1697:bool)  [unwired: 1 in, 1 out]
    n345 = xnode "FPGA I/O Node"() -> ("RMC/DIO40"=w1695:bool)  [unwired: 1 in, 1 out]
    n346 = xnode "FPGA I/O Node"() -> ("RMC/DIO41"=w1693:bool)  [unwired: 1 in, 1 out]
    n347 = xnode "FPGA I/O Node"() -> ("RMC/DIO42"=w1691:bool)  [unwired: 1 in, 1 out]
    n348 = xnode "FPGA I/O Node"() -> ("RMC/DIO43"=w1689:bool)  [unwired: 1 in, 1 out]
    n349 = call "FPGA Debounce Digital.vi"("Input Signal"=w1679, "Cycles to Filter"="Diagnostic Filter") -> ("Output Filtered Signal"=w1698:bool)
    n350 = call "FPGA Debounce Digital.vi"("Input Signal"=w1697, "Cycles to Filter"="Diagnostic Filter") -> ("Output Filtered Signal"=w1696:bool)
    n351 = call "FPGA Debounce Digital.vi"("Input Signal"=w1695, "Cycles to Filter"="Diagnostic Filter") -> ("Output Filtered Signal"=w1694:bool)
    n352 = call "FPGA Debounce Digital.vi"("Input Signal"=w1693, "Cycles to Filter"="Diagnostic Filter") -> ("Output Filtered Signal"=w1692:bool)
    n353 = call "FPGA Debounce Digital.vi"("Input Signal"=w1691, "Cycles to Filter"="Diagnostic Filter") -> ("Output Filtered Signal"=w1690:bool)
    n354 = call "FPGA Debounce Digital.vi"("Input Signal"=w1689, "Cycles to Filter"="Diagnostic Filter") -> ("Output Filtered Signal"=w1688:bool)
    n355 = To Fixed-Point(fixed-point type=fxp<+/-,32,32> 0.0 ("s? t:f"), number="Diagnostic Freq Coeff") -> (fixed-point=w1685:fxp<+/-,32,32>)
    n356 = case shown="\"CMFB\"" "Diagnostic Mode" {
      tunnel: [w1762 w1905 w2151] -> w1758
      tunnel: w1757 -> [_ w1904 w2152]
      tunnel: [w1760 w1903 w2128] -> w1756
      tunnel: w1755 -> [_ w1902 _]
      tunnel: w1754 -> [_ w1901 _]
      tunnel: [w1762 w1895 w2129] -> w1753
      tunnel: w1752 -> [_ w1894 _]
      tunnel: [w1762 w1893 w2129] -> w1751
      tunnel: w1750 -> [_ w1889 w2153]
      tunnel: [w1761 w1888 w2127] -> w1749
      tunnel: w1748 -> [_ w1887 w2148]
      tunnel: [w1762 w1883 w2129] -> w1747
      tunnel: w1746 -> [_ w1882 _]
      tunnel: [w1762 w1881 w2129] -> w1745
      tunnel: w1744 -> [_ w1875 _]
      tunnel: w1743 -> [_ w1874 _]
      tunnel: [w1760 w1873 w2128] -> w1742
      tunnel: w1741 -> [_ w1872 w2149]
      tunnel: [w1762 w1871 w2147] -> w1740
      tunnel: [w1762 w1860 w2143] -> w1739
      tunnel: w1738 -> [_ w1859 w2145]
      tunnel: [w1760 w1858 w2128] -> w1737
      tunnel: w1736 -> [_ w1857 _]
      tunnel: w1735 -> [_ w1856 _]
      tunnel: [w1762 w1850 w2129] -> w1734
      tunnel: w1733 -> [_ w1849 _]
      tunnel: [w1762 w1848 w2129] -> w1732
      tunnel: w1731 -> [_ w1844 w2144]
      tunnel: w1730 -> [_ w1843 w2141]
      tunnel: [w1762 w1839 w2129] -> w1729
      tunnel: w1728 -> [_ w1838 _]
      tunnel: [w1762 w1837 w2129] -> w1727
      tunnel: w1726 -> [_ w1831 _]
      tunnel: w1725 -> [_ w1830 _]
      tunnel: [w1760 w1829 w2128] -> w1724
      tunnel: w1723 -> [_ w1828 w2139]
      tunnel: [w1762 w1827 w2140] -> w1722
      tunnel: [w1762 w1816 w2135] -> w1721
      tunnel: w1720 -> [_ w1815 w2137]
      tunnel: [w1760 w1814 w2128] -> w1719
      tunnel: w1718 -> [_ w1813 _]
      tunnel: w1717 -> [_ w1812 _]
      tunnel: [w1762 w1806 w2129] -> w1716
      tunnel: w1715 -> [_ w1805 _]
      tunnel: [w1762 w1804 w2129] -> w1714
      tunnel: w1713 -> [_ w1800 w2136]
      tunnel: w1712 -> [_ w1799 w2131]
      tunnel: [w1762 w1795 w2129] -> w1711
      tunnel: w1710 -> [_ w1794 _]
      tunnel: [w1762 w1793 w2129] -> w1709
      tunnel: w1708 -> [_ w1787 _]
      tunnel: w1707 -> [_ w1786 _]
      tunnel: [w1760 w1785 w2128] -> w1706
      tunnel: w1705 -> [_ w1784 w2132]
      tunnel: [w1762 w1783 w2130] -> w1704
      tunnel: [w1761 w1777 w2126] -> w1703
      tunnel: [w1761 w1776 w2125] -> w1702
      tunnel: [w1761 w1775 w2124] -> w1701
      tunnel: [w1761 w1774 w2123] -> w1700
      tunnel: [w1761 w1773 w2122] -> w1699
      tunnel: w1698 -> [_ w1772 w2154]
      tunnel: w1696 -> [_ w1771 w2150]
      tunnel: w1694 -> [_ w1770 w2146]
      tunnel: w1692 -> [_ w1769 w2142]
      tunnel: w1690 -> [_ w1768 w2138]
      tunnel: w1688 -> [_ w1767 w2133]
      tunnel: w1685 -> [_ w1766 _]
      tunnel: "Invert Diagnostic" -> [_ w1765 _]
      tunnel: "Diag Max Period (ticks)" -> [_ _ w2134]
      tunnel: [fxp<+/-,28,17>[] [0.0, 0.0, 0.0, 0.0, 0.0, 0.0] w1764 w2121] -> w1680
      frame "None", Default {
        w1760 = FALSE ("Output Filtered Signal")
        w1761 = fxp<+/-,28,17> 0.0 ("AI0")
        w1762 = u32 0 ("f")
      }
      frame "PSA" {
        # "PWM diagnostic code."
        n357 = call "Tick Count2"() -> ("Tick Count(Ticks)"=w1910:u32)
        n358 = call "Tick Count3"() -> ("Tick Count(Ticks)"=w1866:u32)
        n359 = call "Tick Count4"() -> ("Tick Count(Ticks)"=w1865:u32)
        n360 = call "Tick Count5"() -> ("Tick Count(Ticks)"=w1822:u32)
        n361 = call "Tick Count6"() -> ("Tick Count(Ticks)"=w1821:u32)
        n362 = call "Tick Count7"() -> ("Tick Count(Ticks)"=w1778:u32)
        n363 = Greater?(x=w1772, y=w1902) -> (0:w1907:bool)
        n364 = Greater?(x=w1771, y=w1874) -> (0:w1869:bool)
        n365 = Greater?(x=w1770, y=w1857) -> (0:w1862:bool)
        n366 = Greater?(x=w1769, y=w1830) -> (0:w1825:bool)
        n367 = Greater?(x=w1768, y=w1813) -> (0:w1818:bool)
        n368 = Greater?(x=w1767, y=w1786) -> (0:w1781:bool)
        n369 = Subtract(x=w1910, y=w1904) -> (x-y=w1909:u32)
        n370 = Subtract(x=w1866, y=w1872) -> (x-y=w1867:u32)
        n371 = Subtract(x=w1865, y=w1859) -> (x-y=w1864:u32)
        n372 = Subtract(x=w1822, y=w1828) -> (x-y=w1823:u32)
        n373 = Subtract(x=w1821, y=w1815) -> (x-y=w1820:u32)
        n374 = Subtract(x=w1778, y=w1784) -> (x-y=w1779:u32)
        n375 = Less?(x=w1772, y=w1902) -> (x < y?=w1908:bool)
        n376 = Less?(x=w1771, y=w1874) -> (x < y?=w1868:bool)
        n377 = Less?(x=w1770, y=w1857) -> (x < y?=w1863:bool)
        n378 = Less?(x=w1769, y=w1830) -> (x < y?=w1824:bool)
        n379 = Less?(x=w1768, y=w1813) -> (x < y?=w1819:bool)
        n380 = Less?(x=w1767, y=w1786) -> (x < y?=w1780:bool)
        n381 = case shown="True" w1765 {
          tunnel: w1908 -> [w2117 w2119]
          tunnel: w1907 -> [w2116 w2120]
          tunnel: [w2117 w2120] -> w1906
          tunnel: [w2116 w2119] -> w1892
          tunnel: w1772 -> [w2115 w2118]
          tunnel: [w2115 w2118] -> w1903
          frame False {
          }
          frame True {
          }
        }
        n382 = case shown="True" w1765 {
          tunnel: w1868 -> [w2082 w2084]
          tunnel: w1869 -> [w2081 w2085]
          tunnel: [w2082 w2085] -> w1870
          tunnel: [w2081 w2084] -> w1884
          tunnel: w1771 -> [w2080 w2083]
          tunnel: [w2080 w2083] -> w1873
          frame False {
          }
          frame True {
          }
        }
        n383 = case shown="True" w1765 {
          tunnel: w1863 -> [w2047 w2049]
          tunnel: w1862 -> [w2046 w2050]
          tunnel: [w2047 w2050] -> w1861
          tunnel: [w2046 w2049] -> w1847
          tunnel: w1770 -> [w2045 w2048]
          tunnel: [w2045 w2048] -> w1858
          frame False {
          }
          frame True {
          }
        }
        n384 = case shown="True" w1765 {
          tunnel: w1824 -> [w2012 w2014]
          tunnel: w1825 -> [w2011 w2015]
          tunnel: [w2012 w2015] -> w1826
          tunnel: [w2011 w2014] -> w1840
          tunnel: w1769 -> [w2010 w2013]
          tunnel: [w2010 w2013] -> w1829
          frame False {
          }
          frame True {
          }
        }
        n385 = case shown="True" w1765 {
          tunnel: w1819 -> [w1977 w1979]
          tunnel: w1818 -> [w1976 w1980]
          tunnel: [w1977 w1980] -> w1817
          tunnel: [w1976 w1979] -> w1803
          tunnel: w1768 -> [w1975 w1978]
          tunnel: [w1975 w1978] -> w1814
          frame False {
          }
          frame True {
          }
        }
        n386 = case shown="True" w1765 {
          tunnel: w1780 -> [w1942 w1944]
          tunnel: w1781 -> [w1941 w1945]
          tunnel: [w1942 w1945] -> w1782
          tunnel: [w1941 w1944] -> w1796
          tunnel: w1767 -> [w1940 w1943]
          tunnel: [w1940 w1943] -> w1785
          frame False {
          }
          frame True {
          }
        }
        n387 = Select(t=w1909, s=w1906, f=w1901) -> (s? t:f=w1895:u32)
        n388 = Select(t=w1867, s=w1870, f=w1875) -> (s? t:f=w1881:u32)
        n389 = Select(t=w1864, s=w1861, f=w1856) -> (s? t:f=w1850:u32)
        n390 = Select(t=w1823, s=w1826, f=w1831) -> (s? t:f=w1837:u32)
        n391 = Select(t=w1820, s=w1817, f=w1812) -> (s? t:f=w1806:u32)
        n392 = Select(t=w1779, s=w1782, f=w1787) -> (s? t:f=w1793:u32)
        n393 = Select(t=w1910, s=w1892, f=w1904) -> (s? t:f=w1905:u32)
        n394 = Select(t=w1866, s=w1884, f=w1872) -> (s? t:f=w1871:u32)
        n395 = Select(t=w1865, s=w1847, f=w1859) -> (s? t:f=w1860:u32)
        n396 = Select(t=w1822, s=w1840, f=w1828) -> (s? t:f=w1827:u32)
        n397 = Select(t=w1821, s=w1803, f=w1815) -> (s? t:f=w1816:u32)
        n398 = Select(t=w1778, s=w1796, f=w1784) -> (s? t:f=w1783:u32)
        n399 = Select(t=w1895, s=w1892, f=w1894) -> (s? t:f=w1893:u32)
        n400 = Select(t=w1881, s=w1884, f=w1882) -> (s? t:f=w1883:u32)
        n401 = Select(t=w1850, s=w1847, f=w1849) -> (s? t:f=w1848:u32)
        n402 = Select(t=w1837, s=w1840, f=w1838) -> (s? t:f=w1839:u32)
        n403 = Select(t=w1806, s=w1803, f=w1805) -> (s? t:f=w1804:u32)
        n404 = Select(t=w1793, s=w1796, f=w1794) -> (s? t:f=w1795:u32)
        n405 = To Fixed-Point(fixed-point type=fxp<+/-,32,32> 0.0 ("s? t:f"), number=w1893) -> (fixed-point=w1896:fxp<+/-,32,32>)
        n406 = To Fixed-Point(fixed-point type=fxp<+/-,32,32> 0.0 ("s? t:f"), number=w1883) -> (fixed-point=w1880:fxp<+/-,32,32>)
        n407 = To Fixed-Point(fixed-point type=fxp<+/-,32,32> 0.0 ("s? t:f"), number=w1848) -> (fixed-point=w1851:fxp<+/-,32,32>)
        n408 = To Fixed-Point(fixed-point type=fxp<+/-,32,32> 0.0 ("s? t:f"), number=w1839) -> (fixed-point=w1836:fxp<+/-,32,32>)
        n409 = To Fixed-Point(fixed-point type=fxp<+/-,32,32> 0.0 ("s? t:f"), number=w1804) -> (fixed-point=w1807:fxp<+/-,32,32>)
        n410 = To Fixed-Point(fixed-point type=fxp<+/-,32,32> 0.0 ("s? t:f"), number=w1795) -> (fixed-point=w1792:fxp<+/-,32,32>)
        n411 = feedback #17() -> (w1897:bool)  [unwired: 1 in]
        n412 = And(x=w1892, y=w1897) -> (x .and. y?=w1898:bool)
        n413 = feedback #18() -> (w1879:bool)  [unwired: 1 in]
        n414 = And(x=w1884, y=w1879) -> (x .and. y?=w1878:bool)
        n415 = feedback #19() -> (w1852:bool)  [unwired: 1 in]
        n416 = And(x=w1847, y=w1852) -> (x .and. y?=w1853:bool)
        n417 = feedback #20() -> (w1835:bool)  [unwired: 1 in]
        n418 = And(x=w1840, y=w1835) -> (x .and. y?=w1834:bool)
        n419 = feedback #21() -> (w1808:bool)  [unwired: 1 in]
        n420 = And(x=w1803, y=w1808) -> (x .and. y?=w1809:bool)
        n421 = feedback #22() -> (w1791:bool)  [unwired: 1 in]
        n422 = And(x=w1796, y=w1791) -> (x .and. y?=w1790:bool)
        n423 = xnode "High Throughput Divide"("x"=w1896, "y"=w1766, "input valid"=w1898) -> ("x/y"=w1891:fxp<+/-,28,17>, "output valid"=w1890:bool, "ready for input"=w1899:bool)  [unwired: 1 in]
        n424 = feedback-in #17(w1899) -> ()
        n425 = xnode "High Throughput Divide"("x"=w1880, "y"=w1766, "input valid"=w1878) -> ("x/y"=w1885:fxp<+/-,28,17>, "output valid"=w1886:bool, "ready for input"=w1877:bool)  [unwired: 1 in]
        n426 = feedback-in #18(w1877) -> ()
        n427 = xnode "High Throughput Divide"("x"=w1851, "y"=w1766, "input valid"=w1853) -> ("x/y"=w1846:fxp<+/-,28,17>, "output valid"=w1845:bool, "ready for input"=w1854:bool)  [unwired: 1 in]
        n428 = feedback-in #19(w1854) -> ()
        n429 = xnode "High Throughput Divide"("x"=w1836, "y"=w1766, "input valid"=w1834) -> ("x/y"=w1841:fxp<+/-,28,17>, "output valid"=w1842:bool, "ready for input"=w1833:bool)  [unwired: 1 in]
        n430 = feedback-in #20(w1833) -> ()
        n431 = xnode "High Throughput Divide"("x"=w1807, "y"=w1766, "input valid"=w1809) -> ("x/y"=w1802:fxp<+/-,28,17>, "output valid"=w1801:bool, "ready for input"=w1810:bool)  [unwired: 1 in]
        n432 = feedback-in #21(w1810) -> ()
        n433 = xnode "High Throughput Divide"("x"=w1792, "y"=w1766, "input valid"=w1790) -> ("x/y"=w1797:fxp<+/-,28,17>, "output valid"=w1798:bool, "ready for input"=w1789:bool)  [unwired: 1 in]
        n434 = feedback-in #22(w1789) -> ()
        n435 = Select(t=w1891, s=w1890, f=w1889) -> (s? t:f=w1888:fxp<+/-,28,17>)
        n436 = Select(t=w1885, s=w1886, f=w1887) -> (s? t:f=w1777:fxp<+/-,28,17>)
        n437 = Select(t=w1846, s=w1845, f=w1844) -> (s? t:f=w1776:fxp<+/-,28,17>)
        n438 = Select(t=w1841, s=w1842, f=w1843) -> (s? t:f=w1775:fxp<+/-,28,17>)
        n439 = Select(t=w1802, s=w1801, f=w1800) -> (s? t:f=w1774:fxp<+/-,28,17>)
        n440 = Select(t=w1797, s=w1798, f=w1799) -> (s? t:f=w1773:fxp<+/-,28,17>)
        n441 = Build Array(w1888, w1777, w1776, w1775, w1774, w1773) -> (w1764:fxp<+/-,28,17>[])
      }
      frame "CMFB" {
        n442 = disable-structure shown="FPGA_TARGET_CLASS==SBRIO_9627" {
          disable-tunnel: w2154 -> [w2285 _]
          disable-tunnel: w2153 -> [w2284 _]
          disable-tunnel: w2152 -> [w2283 _]
          disable-tunnel: [w2282 _] -> w2151
          disable-tunnel: w2150 -> [w2281 _]
          disable-tunnel: w2149 -> [w2280 _]
          disable-tunnel: w2148 -> [w2279 _]
          disable-tunnel: [w2278 _] -> w2147
          disable-tunnel: w2146 -> [w2277 _]
          disable-tunnel: w2145 -> [w2276 _]
          disable-tunnel: w2144 -> [w2275 _]
          disable-tunnel: [w2274 _] -> w2143
          disable-tunnel: w2142 -> [w2273 _]
          disable-tunnel: w2141 -> [w2272 _]
          disable-tunnel: [w2271 _] -> w2140
          disable-tunnel: w2139 -> [w2270 _]
          disable-tunnel: w2138 -> [w2269 _]
          disable-tunnel: w2137 -> [w2268 _]
          disable-tunnel: w2136 -> [w2267 _]
          disable-tunnel: [w2266 _] -> w2135
          disable-tunnel: w2134 -> [w2265 _]
          disable-tunnel: w2133 -> [w2264 _]
          disable-tunnel: w2132 -> [w2263 _]
          disable-tunnel: w2131 -> [w2262 _]
          disable-tunnel: [w2261 _] -> w2130
          disable-tunnel: [u32 0 _] -> w2129
          disable-tunnel: [FALSE ("Output Filtered Signal") _] -> w2128
          disable-tunnel: [w2258 _] -> w2127
          disable-tunnel: [w2257 _] -> w2126
          disable-tunnel: [w2256 _] -> w2125
          disable-tunnel: [w2255 _] -> w2124
          disable-tunnel: [w2254 _] -> w2123
          disable-tunnel: [w2253 _] -> w2122
          disable-tunnel: [w2252 _] -> w2121
          frame condition #0 (active) {
            w2155 = fxp<+,32,32> 40000000.0 ("x")
            # "CMFB diagnostic code."
            n443 = feedback #23() -> (w2251:bool)  [unwired: 1 in]
            n444 = feedback-in #23(w2285) -> ()
            n445 = feedback #24() -> (w2220:bool)  [unwired: 1 in]
            n446 = feedback-in #24(w2281) -> ()
            n447 = feedback #25() -> (w2219:bool)  [unwired: 1 in]
            n448 = feedback-in #25(w2277) -> ()
            n449 = feedback #26() -> (w2188:bool)  [unwired: 1 in]
            n450 = feedback-in #26(w2273) -> ()
            n451 = feedback #27() -> (w2187:bool)  [unwired: 1 in]
            n452 = feedback-in #27(w2269) -> ()
            n453 = feedback #28() -> (w2156:bool)  [unwired: 1 in]
            n454 = feedback-in #28(w2264) -> ()
            n455 = Increment(x=w2283) -> (x+1=w2248:u32)
            n456 = Increment(x=w2280) -> (x+1=w2223:u32)
            n457 = Increment(x=w2276) -> (x+1=w2216:u32)
            n458 = Increment(x=w2270) -> (x+1=w2191:u32)
            n459 = Increment(x=w2268) -> (x+1=w2184:u32)
            n460 = Increment(x=w2263) -> (x+1=w2159:u32)
            n461 = Greater?(x=w2285, y=w2251) -> (0:w2236:bool)
            n462 = Greater?(x=w2281, y=w2220) -> (0:w2235:bool)
            n463 = Greater?(x=w2277, y=w2219) -> (0:w2204:bool)
            n464 = Greater?(x=w2273, y=w2188) -> (0:w2203:bool)
            n465 = Greater?(x=w2269, y=w2187) -> (0:w2172:bool)
            n466 = Greater?(x=w2264, y=w2156) -> (0:w2171:bool)
            n467 = Greater?(x=w2248, y=w2265) -> (0:w2250:bool)
            n468 = Greater?(x=w2223, y=w2265) -> (0:w2221:bool)
            n469 = Greater?(x=w2216, y=w2265) -> (0:w2218:bool)
            n470 = Greater?(x=w2191, y=w2265) -> (0:w2189:bool)
            n471 = Greater?(x=w2184, y=w2265) -> (0:w2186:bool)
            n472 = Greater?(x=w2159, y=w2265) -> (0:w2157:bool)
            n473 = To Fixed-Point(number=w2248) -> (fixed-point=w2247:fxp<+,32,32>)  [unwired: 1 in]
            n474 = To Fixed-Point(number=w2223) -> (fixed-point=w2224:fxp<+,32,32>)  [unwired: 1 in]
            n475 = To Fixed-Point(number=w2216) -> (fixed-point=w2215:fxp<+,32,32>)  [unwired: 1 in]
            n476 = To Fixed-Point(number=w2191) -> (fixed-point=w2192:fxp<+,32,32>)  [unwired: 1 in]
            n477 = To Fixed-Point(number=w2184) -> (fixed-point=w2183:fxp<+,32,32>)  [unwired: 1 in]
            n478 = To Fixed-Point(number=w2159) -> (fixed-point=w2160:fxp<+,32,32>)  [unwired: 1 in]
            n479 = feedback #29() -> (w2237:bool)  [unwired: 1 in]
            n480 = And(x=w2236, y=w2237) -> (x .and. y?=w2238:bool)
            n481 = feedback #30() -> (w2234:bool)  [unwired: 1 in]
            n482 = And(x=w2235, y=w2234) -> (x .and. y?=w2233:bool)
            n483 = feedback #31() -> (w2205:bool)  [unwired: 1 in]
            n484 = And(x=w2204, y=w2205) -> (x .and. y?=w2206:bool)
            n485 = feedback #32() -> (w2202:bool)  [unwired: 1 in]
            n486 = And(x=w2203, y=w2202) -> (x .and. y?=w2201:bool)
            n487 = feedback #33() -> (w2173:bool)  [unwired: 1 in]
            n488 = And(x=w2172, y=w2173) -> (x .and. y?=w2174:bool)
            n489 = feedback #34() -> (w2170:bool)  [unwired: 1 in]
            n490 = And(x=w2171, y=w2170) -> (x .and. y?=w2169:bool)
            n491 = xnode "High Throughput Divide"("x"=w2155, "y"=w2247, "input valid"=w2238) -> ("x/y"=w2244:fxp<+,28,17>, "output valid"=w2240:bool, "ready for input"=w2239:bool)  [unwired: 1 in]
            n492 = feedback-in #29(w2239) -> ()
            n493 = xnode "High Throughput Divide"("x"=w2155, "y"=w2224, "input valid"=w2233) -> ("x/y"=w2227:fxp<+,28,17>, "output valid"=w2231:bool, "ready for input"=w2232:bool)  [unwired: 1 in]
            n494 = feedback-in #30(w2232) -> ()
            n495 = xnode "High Throughput Divide"("x"=w2155, "y"=w2215, "input valid"=w2206) -> ("x/y"=w2212:fxp<+,28,17>, "output valid"=w2208:bool, "ready for input"=w2207:bool)  [unwired: 1 in]
            n496 = feedback-in #31(w2207) -> ()
            n497 = xnode "High Throughput Divide"("x"=w2155, "y"=w2192, "input valid"=w2201) -> ("x/y"=w2195:fxp<+,28,17>, "output valid"=w2199:bool, "ready for input"=w2200:bool)  [unwired: 1 in]
            n498 = feedback-in #32(w2200) -> ()
            n499 = xnode "High Throughput Divide"("x"=w2155, "y"=w2183, "input valid"=w2174) -> ("x/y"=w2180:fxp<+,28,17>, "output valid"=w2176:bool, "ready for input"=w2175:bool)  [unwired: 1 in]
            n500 = feedback-in #33(w2175) -> ()
            n501 = xnode "High Throughput Divide"("x"=w2155, "y"=w2160, "input valid"=w2169) -> ("x/y"=w2163:fxp<+,28,17>, "output valid"=w2167:bool, "ready for input"=w2168:bool)  [unwired: 1 in]
            n502 = feedback-in #34(w2168) -> ()
            n503 = Select(t=u32 0 ("f"), s=w2240, f=w2248) -> (s? t:f=w2282:u32)
            n504 = Select(t=u32 0 ("f"), s=w2231, f=w2223) -> (s? t:f=w2278:u32)
            n505 = Select(t=u32 0 ("f"), s=w2208, f=w2216) -> (s? t:f=w2274:u32)
            n506 = Select(t=u32 0 ("f"), s=w2199, f=w2191) -> (s? t:f=w2271:u32)
            n507 = Select(t=u32 0 ("f"), s=w2176, f=w2184) -> (s? t:f=w2266:u32)
            n508 = Select(t=u32 0 ("f"), s=w2167, f=w2159) -> (s? t:f=w2261:u32)
            n509 = To Fixed-Point(fixed-point type=fxp<+/-,28,17> 0.0 ("AI0"), number=w2244) -> (fixed-point=w2242:fxp<+/-,28,17>)
            n510 = To Fixed-Point(fixed-point type=fxp<+/-,28,17> 0.0 ("AI0"), number=w2227) -> (fixed-point=w2229:fxp<+/-,28,17>)
            n511 = To Fixed-Point(fixed-point type=fxp<+/-,28,17> 0.0 ("AI0"), number=w2212) -> (fixed-point=w2210:fxp<+/-,28,17>)
            n512 = To Fixed-Point(fixed-point type=fxp<+/-,28,17> 0.0 ("AI0"), number=w2195) -> (fixed-point=w2197:fxp<+/-,28,17>)
            n513 = To Fixed-Point(fixed-point type=fxp<+/-,28,17> 0.0 ("AI0"), number=w2180) -> (fixed-point=w2178:fxp<+/-,28,17>)
            n514 = To Fixed-Point(fixed-point type=fxp<+/-,28,17> 0.0 ("AI0"), number=w2163) -> (fixed-point=w2165:fxp<+/-,28,17>)
            n515 = Or(x=w2250, y=w2240) -> (x .or. y?=w2245:bool)
            n516 = Or(x=w2221, y=w2231) -> (x .or. y?=w2226:bool)
            n517 = Or(x=w2218, y=w2208) -> (x .or. y?=w2213:bool)
            n518 = Or(x=w2189, y=w2199) -> (x .or. y?=w2194:bool)
            n519 = Or(x=w2186, y=w2176) -> (x .or. y?=w2181:bool)
            n520 = Or(x=w2157, y=w2167) -> (x .or. y?=w2162:bool)
            n521 = Select(t=fxp<+/-,28,17> 0.0 ("AI0"), s=w2250, f=w2242) -> (s? t:f=w2246:fxp<+/-,28,17>)
            n522 = Select(t=fxp<+/-,28,17> 0.0 ("AI0"), s=w2221, f=w2229) -> (s? t:f=w2225:fxp<+/-,28,17>)
            n523 = Select(t=fxp<+/-,28,17> 0.0 ("AI0"), s=w2218, f=w2210) -> (s? t:f=w2214:fxp<+/-,28,17>)
            n524 = Select(t=fxp<+/-,28,17> 0.0 ("AI0"), s=w2189, f=w2197) -> (s? t:f=w2193:fxp<+/-,28,17>)
            n525 = Select(t=fxp<+/-,28,17> 0.0 ("AI0"), s=w2186, f=w2178) -> (s? t:f=w2182:fxp<+/-,28,17>)
            n526 = Select(t=fxp<+/-,28,17> 0.0 ("AI0"), s=w2157, f=w2165) -> (s? t:f=w2161:fxp<+/-,28,17>)
            n527 = Select(t=w2246, s=w2245, f=w2284) -> (s? t:f=w2258:fxp<+/-,28,17>)
            n528 = Select(t=w2225, s=w2226, f=w2279) -> (s? t:f=w2257:fxp<+/-,28,17>)
            n529 = Select(t=w2214, s=w2213, f=w2275) -> (s? t:f=w2256:fxp<+/-,28,17>)
            n530 = Select(t=w2193, s=w2194, f=w2272) -> (s? t:f=w2255:fxp<+/-,28,17>)
            n531 = Select(t=w2182, s=w2181, f=w2267) -> (s? t:f=w2254:fxp<+/-,28,17>)
            n532 = Select(t=w2161, s=w2162, f=w2262) -> (s? t:f=w2253:fxp<+/-,28,17>)
            n533 = Build Array(w2258, w2257, w2256, w2255, w2254, w2253) -> (w2252:fxp<+/-,28,17>[])
          }
          frame condition #1 {
          }
        }
      }
    }
    n534 = global write "Diagnostic Global.vi" "Diag_Global"(w1680) -> ()
  }
  n535 = while {
    shift-right: [w2475] -> _
    shift-left: _ -> [w2470]
    stop <- FALSE stop-if-true
    w2462 = refnum<k21> "Signal for Speed"  # FIFO
    # "set at 31.25 kHz"
    n536 = global read "ADC AI Global.vi" "AI16-47"() -> (w2469:fxp<+/-,28,17>[])
    n537 = case shown="1..2500" w2470 {
      tunnel: [fxp<+/-,28,17> -21.0 ("Controller_Current_1 (AI6)") w2515 fxp<+/-,28,17> -22.0 ("Controller_Current_1 (AI6)") w2524 fxp<+/-,28,17> -23.0 ("Controller_Current_1 (AI6)") w2534 fxp<+/-,28,17> -24.0 ("Controller_Current_1 (AI6)") w2543 fxp<+/-,28,17> -25.0 ("Controller_Current_1 (AI6)") w2552 fxp<+/-,28,17> -26.0 ("Controller_Current_1 (AI6)") w2560 fxp<+/-,28,17> -21.5 ("Controller_Current_1 (AI6)") w2569 fxp<+/-,28,17> -22.5 ("Controller_Current_1 (AI6)") w2578 fxp<+/-,28,17> -23.5 ("Controller_Current_1 (AI6)") w2588 fxp<+/-,28,17> -24.5 ("Controller_Current_1 (AI6)") w2597 fxp<+/-,28,17> -25.5 ("Controller_Current_1 (AI6)") w2606 fxp<+/-,28,17> -26.5 ("Controller_Current_1 (AI6)") w2614 fxp<+/-,28,17> -31.0 ("Controller_Current_1 (AI6)")] -> w2466
      tunnel: w2469 -> [_ w2516 _ w2525 _ w2533 _ w2542 _ w2551 _ w2561 _ w2570 _ w2579 _ w2587 _ w2596 _ w2605 _ w2615 _]
      tunnel: [TRUE FALSE TRUE FALSE TRUE FALSE TRUE FALSE TRUE FALSE TRUE FALSE TRUE FALSE TRUE FALSE TRUE FALSE TRUE FALSE TRUE FALSE TRUE FALSE TRUE] -> w2465
      tunnel: "FFT_Amp?" -> [_ w2510 _ w2519 _ w2528 _ w2537 _ w2546 _ w2555 _ w2564 _ w2573 _ w2582 _ w2591 _ w2600 _ w2609 _]
      frame 0, Default {
        # "Start V1"
      }
      frame 1..2500 {
        n538 = Select(t=0 ("index"), s=w2510, f=26) -> (s? t:f=w2512:i32)
        n539 = Index Array(array=w2516, index=w2512) -> (element=w2515:fxp<+/-,28,17>)
      }
      frame 2501 {
        # "Start V2"
      }
      frame 2502..5001 {
        n540 = Select(t=1 ("index"), s=w2519, f=27) -> (s? t:f=w2521:i32)
        n541 = Index Array(array=w2525, index=w2521) -> (element=w2524:fxp<+/-,28,17>)
      }
      frame 5002 {
        # "Start V3"
      }
      frame 5003..7502 {
        n542 = Select(t=2 ("index"), s=w2528, f=28) -> (s? t:f=w2530:i32)
        n543 = Index Array(array=w2533, index=w2530) -> (element=w2534:fxp<+/-,28,17>)
      }
      frame 7503 {
        # "Start V4"
      }
      frame 7504..10003 {
        n544 = Select(t=3 ("index"), s=w2537, f=29) -> (s? t:f=w2539:i32)
        n545 = Index Array(array=w2542, index=w2539) -> (element=w2543:fxp<+/-,28,17>)
      }
      frame 10004 {
        # "Start V5"
      }
      frame 10005..12504 {
        n546 = Select(t=4 ("index"), s=w2546, f=30) -> (s? t:f=w2548:i32)
        n547 = Index Array(array=w2551, index=w2548) -> (element=w2552:fxp<+/-,28,17>)
      }
      frame 12505 {
        # "Start V6"
      }
      frame 12506..15005 {
        n548 = Select(t=5 ("index"), s=w2555, f=31) -> (s? t:f=w2557:i32)
        n549 = Index Array(array=w2561, index=w2557) -> (element=w2560:fxp<+/-,28,17>)
      }
      frame 15006 {
        # "Start V1\nsecond\nread"
      }
      frame 15007..17506 {
        n550 = Select(t=0 ("index"), s=w2564, f=26) -> (s? t:f=w2566:i32)
        n551 = Index Array(array=w2570, index=w2566) -> (element=w2569:fxp<+/-,28,17>)
      }
      frame 17507 {
        # "Start V2\nsecond\nread"
      }
      frame 17508..20007 {
        n552 = Select(t=1 ("index"), s=w2573, f=27) -> (s? t:f=w2575:i32)
        n553 = Index Array(array=w2579, index=w2575) -> (element=w2578:fxp<+/-,28,17>)
      }
      frame 20008 {
        # "Start V3\nSecond\nread"
      }
      frame 20009..22508 {
        n554 = Select(t=2 ("index"), s=w2582, f=28) -> (s? t:f=w2584:i32)
        n555 = Index Array(array=w2587, index=w2584) -> (element=w2588:fxp<+/-,28,17>)
      }
      frame 22509 {
        # "Start V4\nsecond\nread"
      }
      frame 22510..25009 {
        n556 = Select(t=3 ("index"), s=w2591, f=29) -> (s? t:f=w2593:i32)
        n557 = Index Array(array=w2596, index=w2593) -> (element=w2597:fxp<+/-,28,17>)
      }
      frame 25010 {
        # "Start V5\nsecond\nread"
      }
      frame 25011..27510 {
        n558 = Select(t=4 ("index"), s=w2600, f=30) -> (s? t:f=w2602:i32)
        n559 = Index Array(array=w2605, index=w2602) -> (element=w2606:fxp<+/-,28,17>)
      }
      frame 27511 {
        # "Start V6\nsecond\nread"
      }
      frame 27512..30011 {
        n560 = Select(t=5 ("index"), s=w2609, f=31) -> (s? t:f=w2611:i32)
        n561 = Index Array(array=w2615, index=w2611) -> (element=w2614:fxp<+/-,28,17>)
      }
      frame 30012.. {
        # "Hold"
      }
    }
    n562 = xnode "High Throughput Divide"("x"=w2466, "y"=fxp<+,14,14> 13107.0 ("Controller_Current_1 (AI6)")) -> ("x/y"=w2467:fxp<+/-,28,17>)
    n563 = Select(t=w2466, s=w2465, f=w2467) -> (s? t:f=w2464:fxp<+/-,28,17>)
    n564 = To Fixed-Point(fixed-point type=fxp<+/-,25,6> 0.0 ("Controller_Current_1 (AI6)"), number=w2464) -> (fixed-point=w2472:fxp<+/-,25,6>)
    n565 = Increment(x=w2470) -> (x+1=w2476:i32)
    n566 = xnode ("FIFO Write")("Element"=w2472, "Timeout"=0, "FIFO In"=w2462) -> ()  [unwired: 2 out]
    n567 = Greater?(x=w2476, y=31249) -> (0:w2478:bool)
    n568 = call "Wait4"("Count(Ticks)"=u32 1280 ("Count(mSec)")) -> ()  [unwired: 1 out]
    n569 = Select(t=0, s=w2478, f=w2476) -> (s? t:f=w2475:i32)
  }
  n570 = while {
    stop <- FALSE stop-if-true
    n571 = global read "Diagnostic Global.vi" "Diag_Global"() -> (w2619:fxp<+/-,28,17>[])
    n572 = for {
      tunnel: w2619 -> [w2624] mode=indexing
      tunnel: [w2621] -> w2618 mode=indexing
      n573 = Multiply(x=w2624, y=fxp<+/-,28,17> 100.0) -> (x*y=w2622:fxp<+/-,56,34>)
      n574 = To Unsigned Long Integer(number=w2622) -> (unsigned 32bit integer=w2621:u32)
    }
    n575 = global write "Diagnostic Global (U32).vi" "Diag Global (U32)"(w2618) -> ()
  }
  n576 = node-c288(w6) -> ()
  n577 = node-c288(w37) -> ()
